vi "Demo Seq Tester.vi"() -> ()   [LabVIEW 2014]
uses:
  <vilib>/Utility/miscctls.llb/LVRowAndColumnTypeDef.ctl
  TypeDefs/STEP Display.ctl
  Mimico Display/TypeDefs/Mimic Data.ctl
  Mimico Display/TypeDefs/BG Image.ctl
  Mimico Display/TypeDefs/mObject.ctl
  02_SEQ/TypeDefs/Sequence.ctl
  02_SEQ/TypeDefs/STEP.ctl
  02_SEQ/TypeDefs/LogicParsedExpression.ctl
  02_SEQ/TypeDefs/HW InOut MAP.ctl
  02_SEQ/TypeDefs/Program.ctl
  APIs/Data Queue/Control Data Cluster.ctl
  SEQ Monitoring Global Variables.vi
  DO Monitoring Global Variables.vi
  APIs/Message Queue/Enqueue Message (Single).vi
  APIs/Message Queue/WINFAS 2 Message Queue.lvlib
  02_SEQ/SeqLoop.lvlib
  APIs/Data Queue/WINFAS 2 Data Queue.lvlib
  Mimico Display/Mimico Display.lvlib
panel:
  out "Current Prog Name":string caption="Info"
  out "Current Prog Info":string caption="Info"
  in  "MIMIC":bool
  in  "SEC":bool
  in  "HOME":bool
  in  "Tab Control":enum32{"HOME", "SEC", "MIMIC", "MESSAGE"}(tab)=enum."SEC"
  in  "New Cfg":bool
  in  "Open Cfg":bool
  in  "Save Cfg":bool
  in  "New Prog":bool
  in  "Delete Prog":bool
  in  "Config Prog":bool
  in  "I/O Config":bool
  in  "Editor de Programas":i32(listbox)=-1 caption="Secuencia"
  out "Current Sequence":string[][](table)
  in  "Angle":sgl(knob) scale=-720.0..720.0
  in  "Start Sec A-Z":bool
  in  "Start Sec Ciclo":bool
  in  "Tab Control HardW":enum32{"Hw 1", "Hw 2", "Hw 3", "Hw 4", "Hw 5"}(tab)
  in  "Conf In":T1
  in  "Conf In 2":T1
  in  "Conf In 3":T1
  in  "Conf In 4":T1
  in  "Conf In 5":T1
  in  "OutPuts":T2(tab)
  out "View Out":T3
  out "View Out 2":T3
  out "View Out 3":T3
  out "View Out 4":T3
  out "View Out 5":T3
  out "Error":bool
  out "Alarma":bool
  out "Show Main Error&Alarm":string[][](table)
  out "Acept":bool
  out "Alarms Message":string
  out "Error Message":string
  out "Operator Message":string
  out "Mimic":picture
  out "MATH":string
  out "HWAsync 10":string
  out "HWAsync 9":string
  out "HWAsync 8":string
  out "HWAsync 7":string
  out "HWAsync 6":string
  out "HWAsync 5":string
  out "HWAsync 4":string
  out "HWAsync 3":string
  out "HWAsync 2":string
  out "HWAsync 1":string
  out "HWSync 5":string
  out "DO 5":bool[](array[boolean]) caption="DO-HWSync 5 -->"
  out "HWSync 4":string
  out "DO 4":bool[](array[boolean]) caption="DO-HWSync 4 -->"
  out "HWSync 3":string
  out "DO 3":bool[](array[boolean]) caption="DO-HWSync 3 -->"
  out "HWSync 2":string
  out "DO 2":bool[](array[boolean]) caption="DO-HWSync 2 -->"
  out "HWSync 1":string
  out "DO 1":bool[](array[boolean]) caption="DO-HWSync 1 -->"
  in  "MESSAGE":bool
  in  "error in (no error)":errorcluster
  in  "Tab Control 2":enum32{"HOME", "PIC", "TAB"}(tab)=enum."PIC"
  out "Mimic Small":picture
  out "Cond. Avan.":string[][](table)
  # "DEMO - Secuencial"
  # "Lista de Programas de Medición"
  # "Editor de Programas"
  # "Instrucciones: \n1)Utilice los botones de crear o borrar programa para agregar o borrar la referencia a la \"Lista de Programas de Medición\".\n2)Utilice la opción de configuración de programas para editar o configurar el programa previamente creado o cargado.\n3)Utilice la opción de configuración de I/O para configurar todas las entradas y salidas que se deseen usar."
  # "Configuración"
  # "Secuencia de Ciclo de Medición"
  # "Estado"
  # "Encoder"
  # "Mensaje de Operador:"
  # "Alarmas:"
  # "Dispositivos SINCRONOS"
  # "Módulo MATEMATICO"
  # "Dispositivos ASINCRONOS"
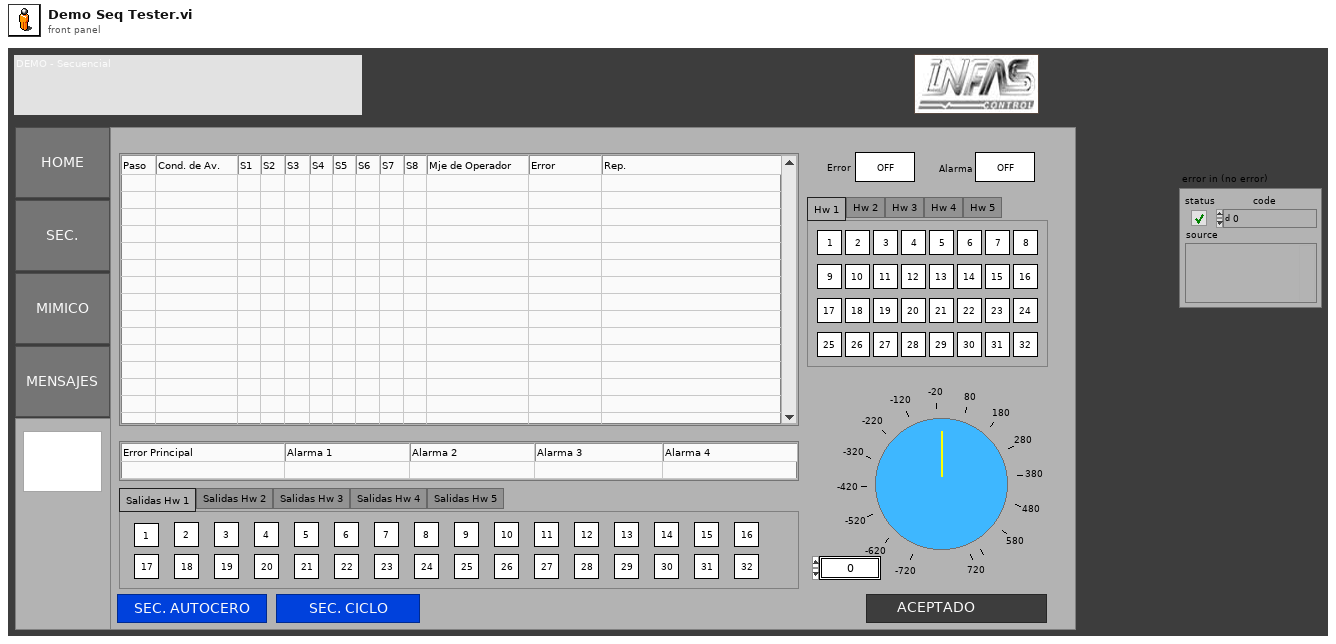
[diagram p1: front panel]
types:
  T1 = cluster{"Boolean 31":bool, "Boolean 2":bool, "Boolean 30":bool, "Boolean 29":bool, "Boolean 28":bool, "Boolean 27":bool, "Boolean 13":bool, "Boolean 14":bool, "Boolean 26":bool, "Boolean 25":bool, "Boolean 24":bool, "Boolean 23":bool, "Boolean 32":bool, "Boolean 1":bool, "Boolean 3":bool, "Boolean 4":bool, "Boolean 5":bool, "Boolean 6":bool, "Boolean 7":bool, "Boolean 8":bool, "Boolean 9":bool, "Boolean 10":bool, "Boolean 11":bool, "Boolean 12":bool, "Boolean 20":bool, "Boolean 18":bool, "Boolean 19":bool, "Boolean 17":bool, "Boolean 16":bool, "Boolean 15":bool, "Boolean 22":bool, "Boolean 21":bool}
  T2 = enum32{"Salidas Hw 1", "Salidas Hw 2", "Salidas Hw 3", "Salidas Hw 4", "Salidas Hw 5"}
  T3 = cluster{"Boolean 36":bool, "Boolean 3":bool, "Boolean 35":bool, "Boolean 34":bool, "Boolean 33":bool, "Boolean 32":bool, "Boolean 16":bool, "Boolean 17":bool, "Boolean 26":bool, "Boolean 25":bool, "Boolean 24":bool, "Boolean 23":bool, "Boolean 37":bool, "Boolean 1":bool, "Boolean 15":bool, "Boolean 4":bool, "Boolean 5":bool, "Boolean 6":bool, "Boolean 7":bool, "Boolean 8":bool, "Boolean 9":bool, "Boolean 10":bool, "Boolean 11":bool, "Boolean 12":bool, "Boolean 38":bool, "Boolean 21":bool, "Boolean 22":bool, "Boolean 20":bool, "Boolean 19":bool, "Boolean 18":bool, "Boolean 40":bool, "Boolean 39":bool}
  T4 = typedef "SeqLoop.lvlib/STEP.ctl" = cluster{"STEP N°":u32, "STEP Switch":cluster{"jump?":bool, "Initial STEP":u32, "Number of STEPs":u32, "Repetitions":u32, "Reset?":bool}, "Outputs":i32[], "STEP Check":cluster{"Advance":T5, "Error ":T5, "Alarm 1":T5, "Alarm 2":T5, "Alarm 3":T5, "Alarm 4":T5}, "Display":cluster{"Mssg Op":string, "Mimic Data":T6}}
  T5 = typedef "SeqLoop.lvlib/LogicParsedExpression.ctl" = cluster{"RPN ":string[], "Variables":string[], "Ctes":string[], "Formula":string, "Message":string}
  T6 = typedef "SeqLoop.lvlib/Mimico Display.lvlib/Mimic Data.ctl" = cluster{"BG Image":T7, "Mimic mObjects":T8[]}
  T7 = typedef "SeqLoop.lvlib/Mimico Display.lvlib/BG Image.ctl" = cluster{"Path":path, "point":cluster{"x":i16, "y":i16}}
  T8 = typedef "SeqLoop.lvlib/Mimico Display.lvlib/mObject.ctl" = cluster{"point":cluster{"x":i16, "y":i16}, "Precision (Digits)":i32, "Visible?":bool, "Ref":string, "Comment":string}
  T9 = typedef "SeqLoop.lvlib/Sequence.ctl" = cluster{"STEPs":T4[], "Main Error&Alarm":cluster{"Main Error":T5, "Main Alarm 1":T5, "Main Alarm 2":T5, "Main Alarm 3":T5, "Main Alarm 4":T5}}
  T10 = cluster{"HWS1":string, "HWS2":string, "HWS3":string, "HWS4":string, "HWS5":string, "MATH":string}
  T11 = enum8{"Enabled", "Disabled", "Disabled and Grayed Out"}
  T12 = typedef "STEP Display.ctl" = cluster{"Mimic Data":T6, "Operator Mssg":string, "Error":cluster{"true?":bool, "Message":string}, "Alarm 1":cluster{"true?":bool, "Message":string}, "Alarm 2":cluster{"true?":bool, "Message":string}, "Alarm 3":cluster{"true?":bool, "Message":string}, "Alarm 4":cluster{"true?":bool, "Message":string}}
  T13 = cluster{"File Direction":path, "Progs Data":variant}
  T14 = typedef "LVRowAndColumnTypeDef.ctl" = cluster{"Row":i32, "Column":i32}
  T15 = typedef "WINFAS 2 Data Queue.lvlib/All Data Queues Cluster.ctl" = cluster{"Queues":cluster{"ACQ HWSync1":refnum<queue>, "ACQ HWSync2":refnum<queue>, "ACQ HWSync3":refnum<queue>, "ACQ HWSync4":refnum<queue>, "ACQ HWSync5":refnum<queue>}, "Notifiers":cluster{"Control":cluster{"CTRL HWSync1":refnum<notifier>, "CTRL HWSync2":refnum<notifier>, "CTRL HWSync3":refnum<notifier>, "CTRL HWSync4":refnum<notifier>, "CTRL HWSync5":refnum<notifier>}, "Acquisition":cluster{"ACQ HWSync1":refnum<notifier>, "ACQ HWSync2":refnum<notifier>, "ACQ HWSync3":refnum<notifier>, "ACQ HWSync4":refnum<notifier>, "ACQ HWSync5":refnum<notifier>}, "Async":cluster{"ACQ HWAsync1":refnum<notifier>, "ACQ HWAsync2":refnum<notifier>, "ACQ HWAsync3":refnum<notifier>, "ACQ HWAsync4":refnum<notifier>, "ACQ HWAsync5":refnum<notifier>, "ACQ HWAsync6":refnum<notifier>, "ACQ HWAsync7":refnum<notifier>, "ACQ HWAsync8":refnum<notifier>, "ACQ HWAsync9":refnum<notifier>, "ACQ HWAsync10":refnum<notifier>}}}
  T16 = typedef "WINFAS 2 Message Queue.lvlib/All Message Queues.ctl" = cluster{"CORE":refnum<queue>, "Event UI":refnum<queue>, "Display UI":refnum<queue>, "MATH":refnum<queue>, "SEQ":refnum<queue>, "DB":refnum<queue>, "ERR":refnum<queue>, "HAL":refnum<queue>, "HWSync1":refnum<queue>, "HWSync2":refnum<queue>, "HWSync3":refnum<queue>, "HWSync4":refnum<queue>, "HWSync5":refnum<queue>, "HWAsync1":refnum<queue>, "HWAsync2":refnum<queue>, "HWAsync3":refnum<queue>, "HWAsync4":refnum<queue>, "HWAsync5":refnum<queue>, "HWAsync6":refnum<queue>, "HWAsync7":refnum<queue>, "HWAsync8":refnum<queue>, "HWAsync9":refnum<queue>, "HWAsync10":refnum<queue>}
  T17 = cluster{"CTRL HWSync1":refnum<notifier>, "CTRL HWSync2":refnum<notifier>, "CTRL HWSync3":refnum<notifier>, "CTRL HWSync4":refnum<notifier>, "CTRL HWSync5":refnum<notifier>}
  T18 = cluster{"File Direction":path, "Progs Data":variant}[]
  T19 = cluster{"Main Error":T5, "Main Alarm 1":T5, "Main Alarm 2":T5, "Main Alarm 3":T5, "Main Alarm 4":T5}
  T20 = enum16{"open", "replace", "create", "open or create", "replace or create", "replace or create with confirmation"}
  T21 = typedef "SeqLoop.lvlib/HW InOut MAP.ctl" = cluster{"Inputs":cluster{"Entrada":i32, "Descripción":string, "Habilitada?":bool}[][], "Outputs":cluster{"Salida":i32, "Descripción":string, "Habilitada?":bool, "Formula":string, "Tipo de Salida":string}[][]}
  T22 = typedef "SeqLoop.lvlib/Program.ctl" = cluster{"Prog. Data":cluster{"Operación":i32, "Pieza":i32, "Descripción":string, "Nombre Programa":string, "Autor":string, "Diseño":string, "Total Meds.:":i32, "Total Meds. Aux.:":i32}, "All Sequences":cluster{"Measurement":T9, "AutoZero":T9}}
  T23 = cluster{cluster{"File Direction":path, "Progs Data":variant}[]}
  T24 = typedef "WINFAS 2 Data Queue.lvlib/Control Data Cluster.ctl" = cluster{"Encoder":sgl, "DI":bool[], "DO":bool[]}
  T25 = cluster{"format string":string, "Measurement Index":i32[]}
  T26 = cluster{"MAX(T) or MIN (F)?":bool, "Mastering TDX Index":i32[]}
  T27 = enum32{"invalid app kind", "Development System", "Run Time System", "Student Edition", "Embedded LabVIEW", "Evaluation", "Custom"}
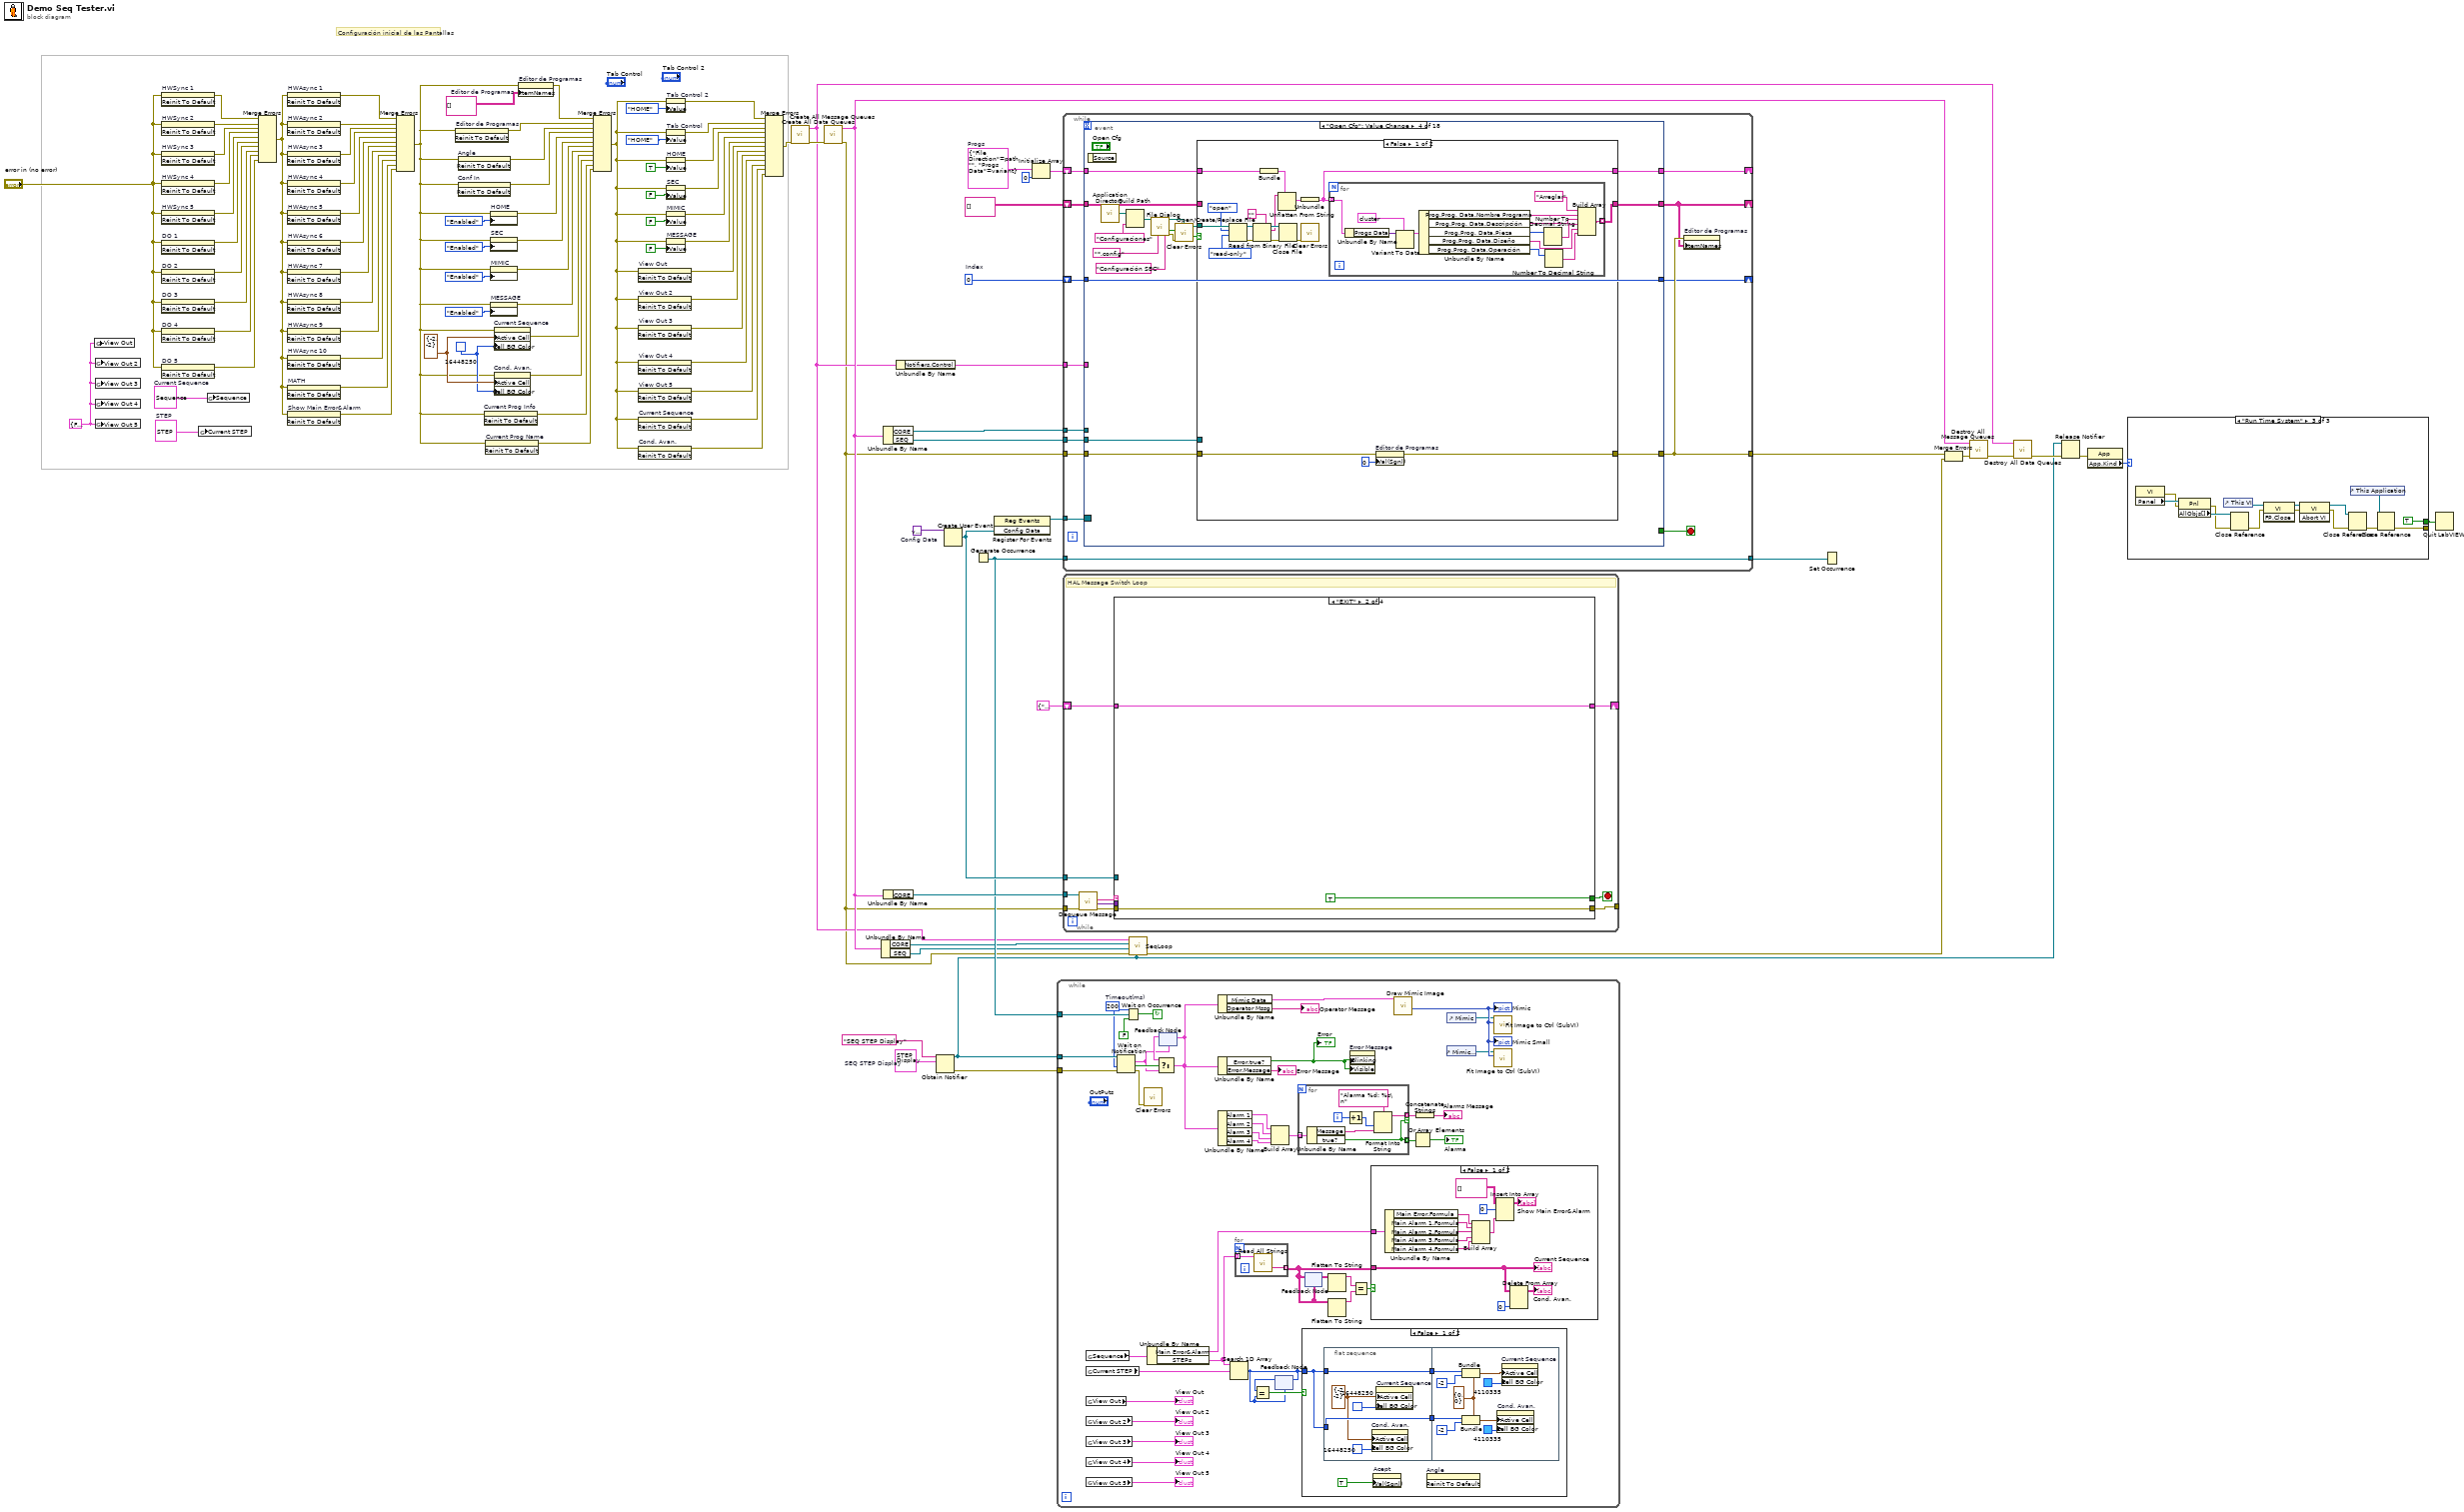
[diagram p0: block diagram]
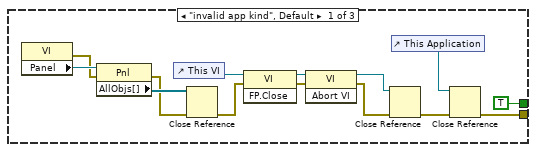
[diagram p4: hidden frame]
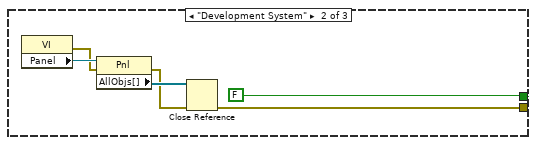
[diagram p5: hidden frame]
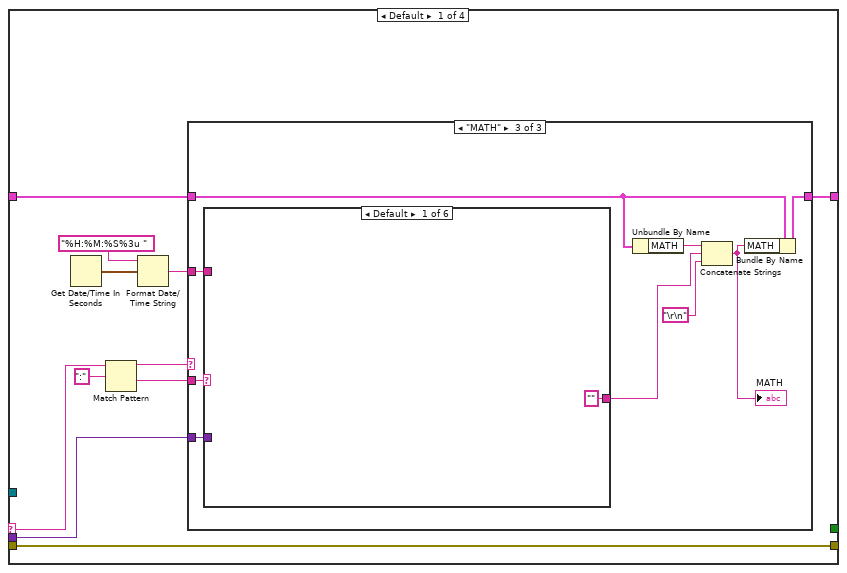
[diagram p6: hidden frame]
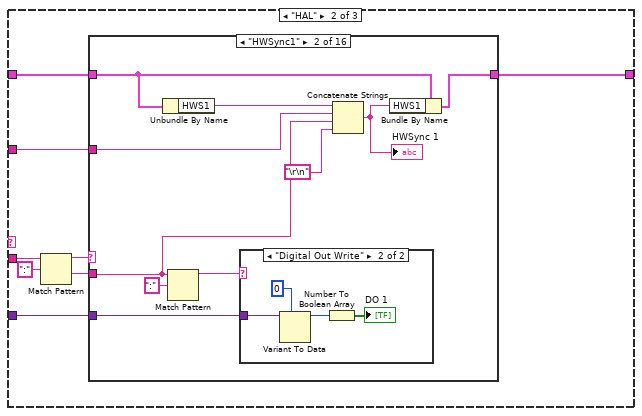
[diagram p8: hidden frame]
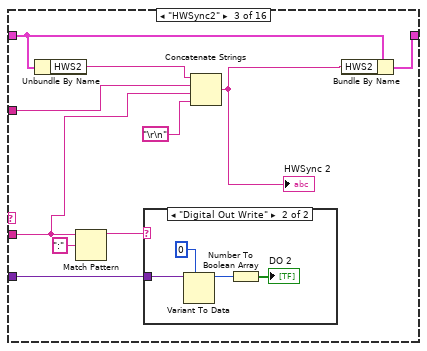
[diagram p11: hidden frame]
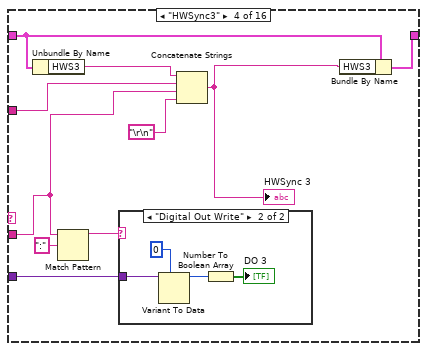
[diagram p13: hidden frame]
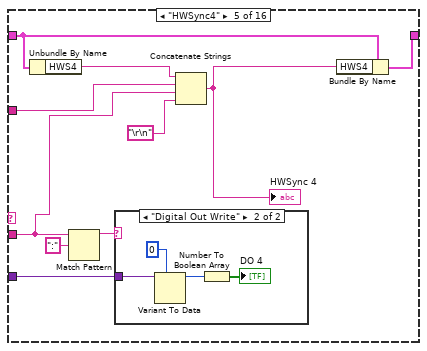
[diagram p15: hidden frame]
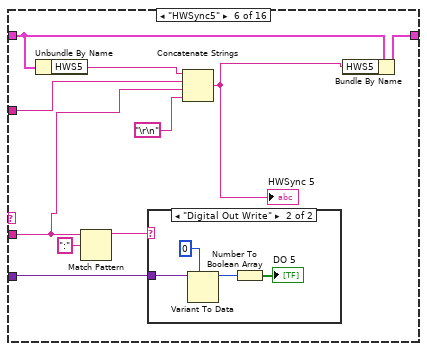
[diagram p17: hidden frame]
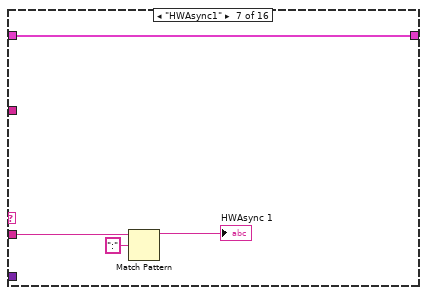
[diagram p19: hidden frame]
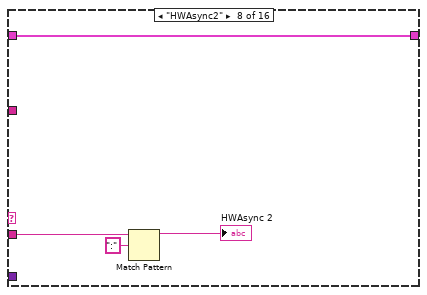
[diagram p20: hidden frame]
diagram:
  w1 = T4 {"STEP N°"=0, "STEP Switch"={"jump?"=FALSE, "Initial STEP"=0, "Number of STEPs"=0, "Repetitions"=0, "Reset?"=FALSE}, "Outputs"=[], "STEP Check"={"Advance"={"RPN "=[], "Variables"=[], "Ctes"=[], "Formula"="", "Message"=""}, "Error "={"RPN "=[], "Variables"=[], "Ctes"=[], "Formula"="", "Message"=""}, "Alarm 1"={"RPN "=[], "Variables"=[], "Ctes"=[], "Formula"="", "Message"=""}, "Alarm 2"={"RPN "=[], "Variables"=[], "Ctes"=[], "Formula"="", "Message"=""}, "Alarm 3"={"RPN "=[], "Variables"=[], "Ctes"=[], "Formula"="", "Message"=""}, "Alarm 4"={"RPN "=[], "Variables"=[], "Ctes"=[], "Formula"="", "Message"=""}}, "Display"={"Mssg Op"="", "Mimic Data"={"BG Image"={"Path"=path "", "point"={"x"=0, "y"=0}}, "Mimic mObjects"=[]}}}  # STEP
  w2 = T3 {"Boolean 36"=FALSE, "Boolean 3"=FALSE, "Boolean 35"=FALSE, "Boolean 34"=FALSE, "Boolean 33"=FALSE, "Boolean 32"=FALSE, "Boolean 16"=FALSE, "Boolean 17"=FALSE, "Boolean 26"=FALSE, "Boolean 25"=FALSE, "Boolean 24"=FALSE, "Boolean 23"=FALSE, "Boolean 37"=FALSE, "Boolean 1"=FALSE, "Boolean 15"=FALSE, "Boolean 4"=FALSE, "Boolean 5"=FALSE, "Boolean 6"=FALSE, "Boolean 7"=FALSE, "Boolean 8"=FALSE, "Boolean 9"=FALSE, "Boolean 10"=FALSE, "Boolean 11"=FALSE, "Boolean 12"=FALSE, "Boolean 38"=FALSE, "Boolean 21"=FALSE, "Boolean 22"=FALSE, "Boolean 20"=FALSE, "Boolean 19"=FALSE, "Boolean 18"=FALSE, "Boolean 40"=FALSE, "Boolean 39"=FALSE} ("View Out")
  w6 = T9 {"STEPs"=[], "Main Error&Alarm"={"Main Error"={"RPN "=[], "Variables"=[], "Ctes"=[], "Formula"="", "Message"=""}, "Main Alarm 1"={"RPN "=[], "Variables"=[], "Ctes"=[], "Formula"="", "Message"=""}, "Main Alarm 2"={"RPN "=[], "Variables"=[], "Ctes"=[], "Formula"="", "Message"=""}, "Main Alarm 3"={"RPN "=[], "Variables"=[], "Ctes"=[], "Formula"="", "Message"=""}, "Main Alarm 4"={"RPN "=[], "Variables"=[], "Ctes"=[], "Formula"="", "Message"=""}}}  # Current Sequence
  w52 = T12 {"Mimic Data"={"BG Image"={"Path"=path "", "point"={"x"=0, "y"=0}}, "Mimic mObjects"=[]}, "Operator Mssg"="", "Error"={"true?"=FALSE, "Message"=""}, "Alarm 1"={"true?"=FALSE, "Message"=""}, "Alarm 2"={"true?"=FALSE, "Message"=""}, "Alarm 3"={"true?"=FALSE, "Message"=""}, "Alarm 4"={"true?"=FALSE, "Message"=""}}  # SEQ STEP Display
  w70 = T13 {"File Direction"=path "", "Progs Data"=variant}  # Progs
  w44 = T14 {"Row"=-2, "Column"=-2} ("Active Cell:Active Cell")
  w43 = u32 16448250
  w73 = string[][] []  # Editor de Programas
  w87 = 0  # Index
  w96 = variant  # Config Data
  # "Configuración inicial de las Pantallas"
  n1 = global write "DO Monitoring Global Variables.vi" "View Out"(w2) -> ()
  n2 = global write "DO Monitoring Global Variables.vi" "View Out 2"(w2) -> ()
  n3 = global write "DO Monitoring Global Variables.vi" "View Out 3"(w2) -> ()
  n4 = global write "DO Monitoring Global Variables.vi" "View Out 4"(w2) -> ()
  n5 = global write "DO Monitoring Global Variables.vi" "View Out 5"(w2) -> ()
  n6 = invoke on="HWSync 1" class="Str" method="Reinit To Default"(error in="error in (no error)") -> (error out=w22:errorcluster)  [unwired: 2 in, 2 out]
  n7 = invoke on="HWSync 2" class="Str" method="Reinit To Default"(error in="error in (no error)") -> (error out=w21:errorcluster)  [unwired: 2 in, 2 out]
  n8 = invoke on="HWSync 3" class="Str" method="Reinit To Default"(error in="error in (no error)") -> (error out=w20:errorcluster)  [unwired: 2 in, 2 out]
  n9 = invoke on="HWSync 4" class="Str" method="Reinit To Default"(error in="error in (no error)") -> (error out=w19:errorcluster)  [unwired: 2 in, 2 out]
  n10 = invoke on="HWSync 5" class="Str" method="Reinit To Default"(error in="error in (no error)") -> (error out=w18:errorcluster)  [unwired: 2 in, 2 out]
  n11 = invoke on="DO 1" class="Arr (strict)" method="Reinit To Default"(error in="error in (no error)") -> (error out=w17:errorcluster)  [unwired: 2 in, 2 out]
  n12 = invoke on="DO 2" class="Arr (strict)" method="Reinit To Default"(error in="error in (no error)") -> (error out=w16:errorcluster)  [unwired: 2 in, 2 out]
  n13 = invoke on="DO 3" class="Arr (strict)" method="Reinit To Default"(error in="error in (no error)") -> (error out=w15:errorcluster)  [unwired: 2 in, 2 out]
  n14 = invoke on="DO 4" class="Arr (strict)" method="Reinit To Default"(error in="error in (no error)") -> (error out=w14:errorcluster)  [unwired: 2 in, 2 out]
  n15 = invoke on="DO 5" class="Arr (strict)" method="Reinit To Default"(error in="error in (no error)") -> (error out=w13:errorcluster)  [unwired: 2 in, 2 out]
  n16 = global write "SEQ Monitoring Global Variables.vi" "Current STEP"(w1) -> ()
  n17 = global write "SEQ Monitoring Global Variables.vi" "Sequence"(w6) -> ()
  n18 = Merge Errors(w22, w21, w20, w19, w18, w17, w16, w15, w14, w13) -> (w4:errorcluster)
  n19 = invoke on="HWAsync 1" class="Str" method="Reinit To Default"(error in=w4) -> (error out=w33:errorcluster)  [unwired: 2 in, 2 out]
  n20 = invoke on="HWAsync 2" class="Str" method="Reinit To Default"(error in=w4) -> (error out=w32:errorcluster)  [unwired: 2 in, 2 out]
  n21 = invoke on="HWAsync 3" class="Str" method="Reinit To Default"(error in=w4) -> (error out=w31:errorcluster)  [unwired: 2 in, 2 out]
  n22 = invoke on="HWAsync 4" class="Str" method="Reinit To Default"(error in=w4) -> (error out=w30:errorcluster)  [unwired: 2 in, 2 out]
  n23 = invoke on="HWAsync 5" class="Str" method="Reinit To Default"(error in=w4) -> (error out=w29:errorcluster)  [unwired: 2 in, 2 out]
  n24 = invoke on="HWAsync 6" class="Str" method="Reinit To Default"(error in=w4) -> (error out=w28:errorcluster)  [unwired: 2 in, 2 out]
  n25 = invoke on="HWAsync 7" class="Str" method="Reinit To Default"(error in=w4) -> (error out=w27:errorcluster)  [unwired: 2 in, 2 out]
  n26 = invoke on="HWAsync 8" class="Str" method="Reinit To Default"(error in=w4) -> (error out=w26:errorcluster)  [unwired: 2 in, 2 out]
  n27 = invoke on="HWAsync 9" class="Str" method="Reinit To Default"(error in=w4) -> (error out=w25:errorcluster)  [unwired: 2 in, 2 out]
  n28 = invoke on="HWAsync 10" class="Str" method="Reinit To Default"(error in=w4) -> (error out=w24:errorcluster)  [unwired: 2 in, 2 out]
  n29 = invoke on="MATH" class="Str" method="Reinit To Default"(error in=w4) -> (error out=w23:errorcluster)  [unwired: 2 in, 2 out]
  n30 = invoke on="Show Main Error&Alarm" class="Tbl (strict)" method="Reinit To Default"(error in=w4) -> (error out=w5:errorcluster)  [unwired: 2 in, 2 out]
  n31 = Merge Errors(w33, w32, w31, w30, w29, w28, w27, w26, w25, w24, w23, w5) -> (w11:errorcluster)
  n32 = invoke on="Editor de Programas" class="MCListbox (strict)" method="Reinit To Default"(error in=w11) -> (error out=w54:errorcluster)  [unwired: 2 in, 2 out]
  n33 = invoke on="Angle" class="Knob (strict)" method="Reinit To Default"(error in=w11) -> (error out=w99:errorcluster)  [unwired: 2 in, 2 out]
  n34 = invoke on="Conf In" class="Clust (strict)" method="Reinit To Default"(error in=w11) -> (error out=w100:errorcluster)  [unwired: 2 in, 2 out]
  n35 = invoke on="Current Prog Info" class="Str" method="Reinit To Default"(error in=w11) -> (error out=w39:errorcluster)  [unwired: 2 in, 2 out]
  n36 = invoke on="Current Prog Name" class="Str" method="Reinit To Default"(error in=w11) -> (error out=w10:errorcluster)  [unwired: 2 in, 2 out]
  n37 = property on="HOME" class="Bool (strict)"(error in=w11, "DisabledEnum"=T11."Enabled" ("Disabled")) -> (error out=w77:errorcluster)  [unwired: 1 in, 1 out]
  n38 = property on="SEC" class="Bool (strict)"(error in=w11, "DisabledEnum"=T11."Enabled" ("Disabled")) -> (error out=w68:errorcluster)  [unwired: 1 in, 1 out]
  n39 = property on="MIMIC" class="Bool (strict)"(error in=w11, "DisabledEnum"=T11."Enabled" ("Disabled")) -> (error out=w67:errorcluster)  [unwired: 1 in, 1 out]
  n40 = property on="MESSAGE" class="Bool (strict)"(error in=w11, "DisabledEnum"=T11."Enabled" ("Disabled")) -> (error out=w45:errorcluster)  [unwired: 1 in, 1 out]
  n41 = property on="Current Sequence" class="Tbl (strict)"(error in=w11, "Active Cell"=w44, "Cell BG Color"=w43) -> (error out=w46:errorcluster)  [unwired: 1 in, 1 out]
  n42 = property on="Cond. Avan." class="Tbl (strict)"(error in=w11, "Active Cell"=w44, "Cell BG Color"=w43) -> (error out=w42:errorcluster)  [unwired: 1 in, 1 out]
  n43 = property on="Editor de Programas" class="MCListbox (strict)"(error in=w11, "ItemNames"=w73) -> (error out=w53:errorcluster)  [unwired: 1 in, 1 out]
  n44 = Merge Errors(w53, w54, w99, w100, w77, w68, w67, w45, w46, w42, w39, w10) -> (w9:errorcluster)
  n45 = invoke on="View Out" class="Clust (strict)" method="Reinit To Default"(error in=w9) -> (error out=w38:errorcluster)  [unwired: 2 in, 2 out]
  n46 = invoke on="View Out 2" class="Clust (strict)" method="Reinit To Default"(error in=w9) -> (error out=w37:errorcluster)  [unwired: 2 in, 2 out]
  n47 = invoke on="View Out 3" class="Clust (strict)" method="Reinit To Default"(error in=w9) -> (error out=w36:errorcluster)  [unwired: 2 in, 2 out]
  n48 = invoke on="View Out 4" class="Clust (strict)" method="Reinit To Default"(error in=w9) -> (error out=w35:errorcluster)  [unwired: 2 in, 2 out]
  n49 = invoke on="View Out 5" class="Clust (strict)" method="Reinit To Default"(error in=w9) -> (error out=w34:errorcluster)  [unwired: 2 in, 2 out]
  n50 = invoke on="Current Sequence" class="Tbl (strict)" method="Reinit To Default"(error in=w9) -> (error out=w8:errorcluster)  [unwired: 2 in, 2 out]
  n51 = invoke on="Cond. Avan." class="Tbl (strict)" method="Reinit To Default"(error in=w9) -> (error out=w7:errorcluster)  [unwired: 2 in, 2 out]
  n52 = property on="Tab Control 2" class="TabCtl (strict)"(error in=w9, "Value"=enum32{"HOME", "PIC", "TAB"}."HOME" ("Tab Control 2")) -> (error out=w41:errorcluster)  [unwired: 1 in, 1 out]
  n53 = property on="Tab Control" class="TabCtl (strict)"(error in=w9, "Value"=enum32{"HOME", "SEC", "MIMIC", "MESSAGE"}."HOME" ("Tab Control")) -> (error out=w76:errorcluster)  [unwired: 1 in, 1 out]
  n54 = property on="HOME" class="Bool (strict)"(error in=w9, "Value"=TRUE ("HOME")) -> (error out=w75:errorcluster)  [unwired: 1 in, 1 out]
  n55 = property on="SEC" class="Bool (strict)"(error in=w9, "Value"=FALSE ("CICLO")) -> (error out=w74:errorcluster)  [unwired: 1 in, 1 out]
  n56 = property on="MIMIC" class="Bool (strict)"(error in=w9, "Value"=FALSE ("CONFIG.")) -> (error out=w66:errorcluster)  [unwired: 1 in, 1 out]
  n57 = property on="MESSAGE" class="Bool (strict)"(error in=w9, "Value"=FALSE ("CONFIG.")) -> (error out=w49:errorcluster)  [unwired: 1 in, 1 out]
  n58 = Merge Errors(w41, w76, w75, w74, w66, w49, w38, w37, w36, w35, w34, w8, w7) -> (w65:errorcluster)
  n59 = call "Create All Data Queues.vi"("Error In"=w65) -> ("Error Out"=w64:errorcluster, "WINFAS 2 Data Queue.lvlib:All Data Queues Cluster"=w57:T15)  [unwired: 9 in]
  n60 = call "Create All Message Queues.vi"("error in (no error)"=w64) -> ("error out"=w56:errorcluster, "Message Queues Out"=w61:T16)  [unwired: 9 in]
  n61 = Unbundle By Name(w61) -> ("CORE"=w59:refnum<queue>, "SEQ"=w58:refnum<queue>)
  n62 = Unbundle By Name(w61) -> ("CORE"=w92:refnum<queue>, "SEQ"=w93:refnum<queue>)
  n63 = Unbundle By Name(w61) -> ("CORE"=w97:refnum<queue>)
  n64 = Unbundle By Name(w57) -> ("Notifiers.Control"=w60:T17)
  n65 = Obtain Notifier(name (unnamed)="SEQ STEP Display", notification data type=w52) -> (notifier out=w51:refnum<notifier>, error out=w83:errorcluster)  [unwired: 2 in, 1 out]
  n66 = Create User Event(user event datatype=w96) -> (user event=w94:refnum<user-event>)  [unwired: 1 in, 1 out]
  n67 = Generate Occurrence() -> (w81:refnum<k4>)
  n68 = register-events(w94) -> (reference out=w95:refnum<event-registration>)  [unwired: 2 in, 1 out]
  n69 = Initialize Array(w70, 0 ("dimension size")) -> (w71:T18)
  n70 = while {
    tunnel: w51 -> [w145]
    tunnel: w83 -> [w140]
    tunnel: w81 -> [w138]
    stop <- w139 continue-if-true
    w136 = 200  # Timeout(ms)
    n71 = global read "SEQ Monitoring Global Variables.vi" "Sequence"() -> (w109:T9)
    n72 = global read "SEQ Monitoring Global Variables.vi" "Current STEP"() -> (w119:T4)
    n73 = global read "DO Monitoring Global Variables.vi" "View Out"() -> (→"View Out":T3)
    n74 = global read "DO Monitoring Global Variables.vi" "View Out 2"() -> (→"View Out 2":T3)
    n75 = global read "DO Monitoring Global Variables.vi" "View Out 3"() -> (→"View Out 3":T3)
    n76 = global read "DO Monitoring Global Variables.vi" "View Out 4"() -> (→"View Out 4":T3)
    n77 = global read "DO Monitoring Global Variables.vi" "View Out 5"() -> (→"View Out 5":T3)
    n78 = Wait on Notification(notifier=w145, timeout in ms (-1)=w136, error in (no error)=w140) -> (notification=w137:T12, timed out?=w144:bool, error out=w142:errorcluster)  [unwired: 1 in, 1 out]
    n79 = Wait on Occurrence(1:FALSE ("ignore previous (T)"), 2:w138, 3:w136) -> (0:w139:bool)
    n80 = call <vilib>:"Clear Errors.vi"("error in (no error)"=w142) -> ()  [unwired: 5 in, 2 out]
    n81 = Unbundle By Name(w109) -> ("Main Error&Alarm"=w102:T19, "STEPs"=w108:T4[])
    n82 = feedback #1(w137) -> (w143:T12)
    n83 = Select(t=w143, s=w144, f=w137) -> (s? t:f=w129:T12)
    n84 = feedback-in #1(w129) -> ()
    n85 = Unbundle By Name(w129) -> ("Mimic Data"=w132:T6, "Operator Mssg"=→"Operator Message":string)
    n86 = Unbundle By Name(w129) -> ("Error.true?"=w110:bool, "Error.Message"=→"Error Message":string)
    "Error" <- w110
    n87 = Unbundle By Name(w129) -> ("Alarm 1"=w128:cluster{"true?":bool, "Message":string}, "Alarm 2"=w127:cluster{"true?":bool, "Message":string}, "Alarm 3"=w126:cluster{"true?":bool, "Message":string}, "Alarm 4"=w125:cluster{"true?":bool, "Message":string})
    n88 = Search 1D Array(1D array=w108, element=w119) -> (index of element=w118:i32)  [unwired: 1 in]
    n89 = for {
      tunnel: w108 -> [w178] mode=indexing
      tunnel: [w177] -> w103 mode=indexing
      n90 = call "Read All Strings.vi"("STEP in"=w178) -> ("All Strings"=w177:string[])  [unwired: 8 in, 2 out]
    }
    n91 = Build Array(w128, w127, w126, w125) -> (w124:cluster{"true?":bool, "Message":string}[])
    n92 = feedback #2(w118) -> (w121:i32)
    n93 = Equal?(x=w121, y=w118) -> (x = y?=w120:bool)
    n94 = feedback-in #2(w118) -> ()
    n95 = for {
      tunnel: w124 -> [w185] mode=indexing
      tunnel: [w180] -> w123 mode=indexing if=w179
      tunnel: [w179] -> w112 mode=indexing
      i -> [w183]
      n96 = Unbundle By Name(w185) -> ("Message"=w181:string, "true?"=w179:bool)
      n97 = Increment(x=w183) -> (x+1=w182:i32)
      n98 = Format Into String(format string="Alarma %d: %s\n", w182, w181) -> (resulting string=w180:string)  [unwired: 2 in, 1 out]
    }
    n99 = case shown="False" w120 {
      tunnel: w118 -> [w160 _]
      frame False {
        n100 = flat-sequence {
          tunnel: w160 -> [w167]
          tunnel: [w167] -> w162
          tunnel: [w164] -> w161
          tunnel: w160 -> [w164]
          tunnel: w162 -> [w173]
          tunnel: w161 -> [w172]
          frame #0 {
            w163 = T14 {"Row"=-2, "Column"=-2} ("Active Cell:Active Cell")
            n101 = property on="Cond. Avan." class="Tbl (strict)"("Active Cell"=w163, "Cell BG Color"=u32 16448250) -> ()  [unwired: 2 in, 2 out]
            n102 = property on="Current Sequence" class="Tbl (strict)"("Active Cell"=w163, "Cell BG Color"=u32 16448250) -> ()  [unwired: 2 in, 2 out]
          }
          frame #1 {
            w168 = cluster{i32, "Row":i32} {0, "Row"=0} ("output cluster")
            n103 = Bundle(cluster=w168, w173, "Row"=-2) -> (w175:cluster{i32, "Row":i32})
            n104 = Bundle(cluster=w168, w172, "Row"=-2) -> (w170:cluster{i32, "Row":i32})
            n105 = property on="Cond. Avan." class="Tbl (strict)"("Active Cell"=w170, "Cell BG Color"=u32 4110335) -> ()  [unwired: 2 in, 2 out]
            n106 = property on="Current Sequence" class="Tbl (strict)"("Active Cell"=w175, "Cell BG Color"=u32 4110335) -> ()  [unwired: 2 in, 2 out]
          }
        }
        n107 = property on="Acept" class="Bool"("Val(Sgnl)"=TRUE) -> ()  [unwired: 2 in, 2 out]
        n108 = invoke on="Angle" class="Knob (strict)" method="Reinit To Default"() -> ()  [unwired: 3 in, 3 out]
      }
      frame True {
      }
    }
    n109 = feedback #3(w103) -> (w107:string[][])
    n110 = feedback-in #3(w103) -> ()
    n111 = Flatten To String(anything=w107) -> (data string=w106:string)  [unwired: 3 in, 2 out]
    n112 = Flatten To String(anything=w103) -> (data string=w105:string)  [unwired: 3 in, 2 out]
    n113 = property on="Error Message" class="Str"("Blinking"=w110, "Visible"=w110) -> ()  [unwired: 2 in, 2 out]
    n114 = Equal?(x=w106, y=w105) -> (x = y?=w104:bool)
    n115 = case shown="False" w104 {
      tunnel: w103 -> [w156 _]
      tunnel: w102 -> [w152 _]
      frame False {
        n116 = Unbundle By Name(w152) -> ("Main Error.Formula"=w150:string, "Main Alarm 1.Formula"=w149:string, "Main Alarm 2.Formula"=w151:string, "Main Alarm 3.Formula"=w148:string, "Main Alarm 4.Formula"=w147:string)
        n117 = Build Array(w150, w149, w151, w148, w147) -> (w146:string[])
        n118 = Insert Into Array(array=string[][] [] ("Show Main Error&Alarm 2"), index (row)=0, new element=w146) -> (→"Show Main Error&Alarm":string[][])  [unwired: 1 in]
        n119 = Delete From Array(array=w156, index (col)=0 ("disabled index (col)")) -> (array with subset deleted=→"Cond. Avan.":string[][])  [unwired: 2 in, 1 out]
        "Current Sequence" <- w156
      }
      frame True {
      }
    }
    n120 = call "Draw Mimic Image.vi"("Mimic Data in"=w132) -> ("Mimic Picture"=w135:picture)  [unwired: 10 in]
    "Mimic" <- w135
    "Mimic Small" <- w135
    n121 = Or Array Elements(Boolean array=w112) -> (logical OR=→"Alarma":bool)
    n122 = Concatenate Strings(w123) -> (→"Alarms Message":string)
    n123 = control-ref of="Mimic"() -> (w134:refnum<vi>)
    n124 = control-ref of="Mimic Small"() -> (w133:refnum<vi>)
    n125 = call "Fit Image to Ctrl (SubVI).vi"("picture in"=w135, "Picture ref in"=w134) -> ()  [unwired: 10 in]
    n126 = call "Fit Image to Ctrl (SubVI).vi"("picture in"=w135, "Picture ref in"=w133) -> ()  [unwired: 10 in]
  }
  n127 = while {
    tunnel: w56 -> [w199]
    tunnel: [w193] -> w101
    tunnel: w95 -> [w197]
    tunnel: w93 -> [w196]
    tunnel: w92 -> [w195]
    shift-right: [w192] -> _
    shift-left: w87 -> [w194]
    tunnel: w81 -> [w191]
    tunnel: [w191] -> w82
    shift-right: [w189] -> _
    shift-left: w71 -> [w190]
    shift-right: [w187] -> _
    shift-left: string[][] [] -> [w188]
    tunnel: w60 -> [w186]
    stop <- w198 stop-if-true
    n128 = event shown="[3] \"Open Cfg\": Value Change" {
      selector: w197 -> [_ _ _ _ _ _ _ _ _ _ _ _ _ _ _ _ _ _]
      dyn-events: _ -> [_ _ _ _ _ _ _ _ _ _ _ _ _ _ _ _ _ _]
      timeout: _ -> [_ _ _ _ _ _ _ _ _ _ _ _ _ _ _ _ _ _]
      tunnel: w199 -> [w216 w230 w252 w291 w338 w360 w390 w412 w435 w460 w482 w497 w504 w527 w548 w569 w610 w638]
      tunnel: [w221 w226 w268 w289 w337 w385 w406 w434 w454 w467 w480 w498 w518 w525 w546 w567 w604 w636] -> w193
      tunnel: [_ _ _ _ _ _ _ _ _ _ _ _ _ _ _ _ _ TRUE ("Discard?")] -> w198
      tunnel: w196 -> [w223 _ w253 w292 _ w362 _ _ _ _ w483 w496 _ w544 w564 _ _ w634]
      tunnel: w195 -> [_ _ _ _ _ _ _ _ _ _ _ _ _ w526 w547 _ _ w635]
      tunnel: ["Editor de Programas" w233 w256 w302 _ w369 w402 w413 w452 _ w485 w493 w513 w542 w563 w566 w628 w633] -> w192
      tunnel: w194 -> [_ w235 w259 w302 _ w363 w402 w413 w452 _ w485 w493 w513 w542 w563 w566 w628 w633]
      tunnel: w190 -> [w225 w229 w261 w293 w340 w364 w401 w427 w448 w479 w484 w495 w520 w541 w562 w572 w630 w632]
      tunnel: [w225 w228 w260 w290 w340 w370 w401 w427 w448 w479 w484 w495 w519 w541 w562 w572 w630 w632] -> w189
      tunnel: w188 -> [w200 w232 w258 w287 w339 w386 w400 w414 w444 w478 w489 w494 w516 w540 w561 w571 w629 w631]
      tunnel: [w200 w231 w257 w288 w339 w387 w400 w414 w444 w478 w489 w494 w515 w540 w561 w571 w629 w631] -> w187
      tunnel: w186 -> [_ _ _ _ _ _ _ _ _ _ _ _ _ _ _ _ w603 _]
      event "Editor de Programas": Value Change {
        w215 = T14 {"Row"=-2, "Column"=-2} ("Active Cell:Active Cell")
        w214 = u32 16448250
        n129 = event-data() -> ()  [unwired: 1 in, 1 out]
        n130 = property on="Current Sequence" class="Tbl (strict)"(error in=w216, "Active Cell"=w215, "Cell BG Color"=w214) -> (error out=w212:errorcluster)  [unwired: 1 in, 1 out]
        n131 = property on="Cond. Avan." class="Tbl (strict)"(error in=w216, "Active Cell"=w215, "Cell BG Color"=w214) -> (error out=w213:errorcluster)  [unwired: 1 in, 1 out]
        n132 = Index Array(array=w200, index (row) #1="Editor de Programas", index (col) #1=1 ("disabled index (col)"), index (row) #2="Editor de Programas", index (col) #2=0 ("disabled index (col)"), index (row) #3="Editor de Programas", index (col) #3=2 ("index (row)"), index (row) #4="Editor de Programas", index (col) #4=6 ("index (col)")) -> (element #1=w203:string, element #2=w210:string, element #3=w209:string, element #4=w208:string)
        n133 = Merge Errors(w212, w213) -> (w211:errorcluster)
        n134 = Index Array(array=w225, index="Editor de Programas") -> (element=w222:T13)
        n135 = Unbundle By Name(w222) -> ("Progs Data"=w217:variant)
        n136 = Concatenate Strings("Nombre Programa: ", w203) -> (→"Current Prog Name":string)
        n137 = call-poly "Enqueue Message.vi"("error in (no error)"=w211, "Message Data"=w217, "Message"="Config:Set" ("Cmd String"), "Message Queue"=w223) -> ("error out"=w221:errorcluster)  [unwired: 6 in, 1 out]
        n138 = Format Into String(format string="COD. Prog. : %s - Descripción: %s - Tipo de Prog.: %s", w210, w209, w208) -> (resulting string=→"Current Prog Info":string)  [unwired: 2 in, 1 out]
      }
      event "Delete Prog": Value Change {
        n139 = event-data() -> ()  [unwired: 1 in, 1 out]
        n140 = Increment(x=w235) -> (x+1=w236:i32)
        n141 = Number To Decimal String(number=w236) -> (decimal integer string=w238:string)  [unwired: 1 in]
        n142 = Concatenate Strings("Desea Borrar el elemento: " ("message"), w238) -> (w237:string)
        n143 = Two Button Dialog(message=w237) -> (T button?=w234:bool)  [unwired: 2 in]
        n144 = case shown="False" w234 {
          tunnel: [w243 w249] -> w231
          tunnel: w232 -> [w243 w248]
          tunnel: w235 -> [w242 w244]
          tunnel: w230 -> [w241 w247]
          tunnel: [w241 w247] -> w227
          tunnel: [w242 w244] -> w233
          tunnel: w229 -> [w240 w246]
          tunnel: [w240 w245] -> w228
          frame False {
          }
          frame True {
            n145 = Delete From Array(array=w246, index=w244) -> (array with subset deleted=w245:T18)  [unwired: 1 in, 1 out]
            n146 = Delete From Array(array=w248, index (row)=w244) -> (array with subset deleted=w249:string[][])  [unwired: 2 in, 1 out]
          }
        }
        n147 = invoke on="Current Prog Info" class="Str" method="Reinit To Default"(error in=w227) -> (error out=w226:errorcluster)  [unwired: 2 in, 2 out]
      }
      event "New Cfg": Value Change {
        w255 = T13 {"File Direction"=path "", "Progs Data"=variant}  # Progs
        n148 = event-data() -> ()  [unwired: 1 in, 1 out]
        n149 = Initialize Array(w255, 15 ("dimension size")) -> (w264:T18)
        n150 = Flatten To String(anything=w264) -> (data string=w266:string)  [unwired: 3 in, 2 out]
        n151 = Flatten To String(anything=w261) -> (data string=w265:string)  [unwired: 3 in, 2 out]
        n152 = Not Equal?(x=w265, y=w266) -> (x != y?=w267:bool)
        n153 = case "Algún Prog cargado?" shown="True" w267 {
          tunnel: [TRUE ("T button?") w273] -> w262
          frame False {
          }
          frame True {
            n154 = Two Button Dialog(message="Desea crear una nueva lista de Programas?\n(Se descargarán todos los Programas cargados)") -> (T button?=w273:bool)  [unwired: 2 in]
          }
        }
        n155 = case shown="False" w262 {
          tunnel: [w277 w285] -> w260
          tunnel: w261 -> [w277 _]
          tunnel: w259 -> [w275 _]
          tunnel: w258 -> [w276 _]
          tunnel: [w276 string[][] []] -> w257
          tunnel: [w275 0 ("Index")] -> w256
          tunnel: w253 -> [_ w280]
          tunnel: w252 -> [w274 w279]
          tunnel: [w274 w278] -> w250
          frame False {
          }
          frame True {
            w282 = T13 {"File Direction"=path "", "Progs Data"=variant}  # Progs
            n156 = call-poly "Enqueue Message.vi"("error in (no error)"=w279, "Message"="INIT" ("Cmd String"), "Message Queue"=w280) -> ("error out"=w278:errorcluster)  [unwired: 7 in, 1 out]
            n157 = Initialize Array(w282, 0 ("dimension size")) -> (w285:T18)
          }
        }
        n158 = invoke on="Angle" class="Knob (strict)" method="Reinit To Default"(error in=w250) -> (error out=w269:errorcluster)  [unwired: 2 in, 2 out]
        n159 = invoke on="Conf In" class="Clust (strict)" method="Reinit To Default"(error in=w250) -> (error out=w270:errorcluster)  [unwired: 2 in, 2 out]
        n160 = invoke on="Current Sequence" class="Tbl (strict)" method="Reinit To Default"(error in=w250) -> (error out=w254:errorcluster)  [unwired: 2 in, 2 out]
        n161 = invoke on="Cond. Avan." class="Tbl (strict)" method="Reinit To Default"(error in=w250) -> (error out=w251:errorcluster)  [unwired: 2 in, 2 out]
        n162 = Merge Errors(w269, w270, w254, w251) -> (w268:errorcluster)
      }
      event "Open Cfg": Value Change {
        n163 = event-data() -> ()  [unwired: 1 in, 1 out]
        n164 = call <vilib>:"Application Directory.vi"() -> ("Application Directory"=w298:path)
        n165 = Build Path(base path=w298, name or relative path="Configuraciones") -> (appended path=w299:path)
        n166 = call "File Dialog"("start path"=w299, "pattern (all files)"="*.config", "pattern label"="Configuración SEC") -> ("selected path"=w294:path, "cancelled"=w301:bool, "error out"=w297:errorcluster)  [unwired: 9 in, 1 out]
        n167 = call <vilib>:"Clear Errors.vi"("error in (no error)"=w297) -> ()  [unwired: 5 in, 2 out]
        n168 = case shown="False" w301 {
          tunnel: w294 -> [w320 _]
          tunnel: w293 -> [w307 w336]
          tunnel: [w306 w336] -> w290
          tunnel: w292 -> [_ _]
          tunnel: w291 -> [w304 w335]
          tunnel: [w303 w335] -> w289
          tunnel: [w308 w334] -> w288
          tunnel: w287 -> [_ w334]
          frame False {
            n169 = Open/Create/Replace File(file path (use dialog)=w320, operation (0:open)=T20."open", access (0:read/write)=enum16{"read/write", "read-only", "write-only"}."read-only") -> (refnum out=w318:refnum<file>, error out=w316:errorcluster)  [unwired: 3 in, 1 out]
            n170 = Read from Binary File(5:"", 8:w316, 11:w318) -> (0:w315:errorcluster, 2:w313:string, 3:w317:refnum<file>)  [unwired: 3 in, 1 out]
            n171 = Bundle(w307) -> (w312:T23)  [unwired: 1 in]
            n172 = Unflatten From String(type=w312, binary string=w313) -> (value=w311:T23)  [unwired: 3 in, 2 out]
            n173 = Close File(refnum=w317, error in=w315) -> (error out=w314:errorcluster)  [unwired: 1 out]
            n174 = Unbundle(w311) -> (w306:T18)
            n175 = call <vilib>:"Clear Errors.vi"("error in (no error)"=w314) -> ()  [unwired: 5 in, 2 out]
            n176 = for {
              tunnel: w306 -> [w333] mode=indexing
              tunnel: [w324] -> w308 mode=indexing
              n177 = Unbundle By Name(w333) -> ("Progs Data"=w323:variant)
              n178 = Variant To Data(type=cluster{"I/O Map":T21, "Prog":T22} {"I/O Map"={"Inputs"=[], "Outputs"=[]}, "Prog"={"Prog. Data"={"Operación"=0, "Pieza"=0, "Descripción"="", "Nombre Programa"="", "Autor"="", "Diseño"="", "Total Meds.:"=0, "Total Meds. Aux.:"=0}, "All Sequences"={"Measurement"={"STEPs"=[], "Main Error&Alarm"={"Main Error"={"RPN "=[], "Variables"=[], "Ctes"=[], "Formula"="", "Message"=""}, "Main Alarm 1"={"RPN "=[], "Variables"=[], "Ctes"=[], "Formula"="", "Message"=""}, "Main Alarm 2"={"RPN "=[], "Variables"=[], "Ctes"=[], "Formula"="", "Message"=""}, "Main Alarm 3"={"RPN "=[], "Variables"=[], "Ctes"=[], "Formula"="", "Message"=""}, "Main Alarm 4"={"RPN "=[], "Variables"=[], "Ctes"=[], "Formula"="", "Message"=""}}}, "AutoZero"={"STEPs"=[], "Main Error&Alarm"={"Main Error"={"RPN "=[], "Variables"=[], "Ctes"=[], "Formula"="", "Message"=""}, "Main Alarm 1"={"RPN "=[], "Variables"=[], "Ctes"=[], "Formula"="", "Message"=""}, "Main Alarm 2"={"RPN "=[], "Variables"=[], "Ctes"=[], "Formula"="", "Message"=""}, "Main Alarm 3"={"RPN "=[], "Variables"=[], "Ctes"=[], "Formula"="", "Message"=""}, "Main Alarm 4"={"RPN "=[], "Variables"=[], "Ctes"=[], "Formula"="", "Message"=""}}}}}}, Variant=w323) -> (data=w325:cluster{"I/O Map":T21, "Prog":T22})  [unwired: 1 in, 1 out]
              n179 = Unbundle By Name(w325) -> ("Prog.Prog. Data.Nombre Programa"=w326:string, "Prog.Prog. Data.Descripción"=w327:string, "Prog.Prog. Data.Pieza"=w328:i32, "Prog.Prog. Data.Diseño"=w330:string, "Prog.Prog. Data.Operación"=w331:i32)
              n180 = Number To Decimal String(number=w328) -> (decimal integer string=w329:string)  [unwired: 1 in]
              n181 = Number To Decimal String(number=w331) -> (decimal integer string=w332:string)  [unwired: 1 in]
              n182 = Build Array("Arreglar" ("element"), w326, w327, w329, w330, w332) -> (w324:string[])
            }
            n183 = property on="Editor de Programas" class="MCListbox (strict)"(error in=w304, "Val(Sgnl)"=0 ("Value (Signaling)")) -> (error out=w303:errorcluster)  [unwired: 1 in, 1 out]
          }
          frame True {
          }
        }
      }
      event "Save Cfg": Value Change {
        n184 = event-data() -> ()  [unwired: 1 in, 6 out]
        n185 = call <vilib>:"Application Directory.vi"() -> ("Application Directory"=w346:path)
        n186 = Build Path(base path=w346, name or relative path="Configuraciones") -> (appended path=w348:path)
        n187 = Bundle(w340) -> (w349:T23)  [unwired: 1 in]
        n188 = call "File Dialog2"("start path"=w348, "pattern (all files)"="*.config", "pattern label"="Configuración SEC") -> ("selected path"=w341:path, "cancelled"=w344:bool, "error out"=w345:errorcluster)  [unwired: 9 in, 1 out]
        n189 = Flatten To String(anything=w349, error in (no error)=w338) -> (data string=w350:string, error out=w337:errorcluster)  [unwired: 2 in, 1 out]
        n190 = call <vilib>:"Clear Errors.vi"("error in (no error)"=w345) -> ()  [unwired: 5 in, 2 out]
        n191 = case shown="True" w344 {
          tunnel: w350 -> [w358 _]
          tunnel: w341 -> [w354 _]
          frame False {
            n192 = Open/Create/Replace File(file path (use dialog)=w354, operation (0:open)=T20."open or create", access (0:read/write)=enum16{"read/write", "read-only", "write-only"}."write-only") -> (refnum out=w355:refnum<file>, error out=w352:errorcluster)  [unwired: 3 in, 1 out]
            n193 = Write to Binary File(file (use dialog)=w355, data=w358, error in=w352) -> (refnum out=w353:refnum<file>, error out=w351:errorcluster)  [unwired: 3 in, 1 out]
            n194 = Close File(refnum=w353, error in=w351) -> ()  [unwired: 2 out]
          }
          frame True {
          }
        }
      }
      event "New Prog": Value Change {
        w366 = T13 {"File Direction"=path "", "Progs Data"=variant}  # Progs
        n195 = event-data() -> ()  [unwired: 1 in, 1 out]
        n196 = Matrix Size(0:w386) -> (1:w369:i32)  [unwired: 1 out]
        n197 = Number To Decimal String(number=w369) -> (decimal integer string=w377:string)  [unwired: 1 in]
        n198 = Index Array(array=w364, index=w363) -> (element=w359:T13)
        n199 = Concatenate Strings("Cod. Prog. ", w377) -> (w383:string)
        n200 = Concatenate Strings("Nombre Programa ", w377) -> (w382:string)
        n201 = Concatenate Strings("Descripción ", w377) -> (w381:string)
        n202 = Concatenate Strings("Pieza ", w377) -> (w380:string)
        n203 = Concatenate Strings("Diseño ", w377) -> (w379:string)
        n204 = Concatenate Strings("Operación ", w377) -> (w378:string)
        n205 = Build Array(w383, w382, w381, w380, w379, w378, "CAP" ("element")) -> (w384:string[])
        n206 = To Variant(anything=w359) -> (Variant=w365:variant)
        n207 = call-poly "Enqueue Message.vi"("error in (no error)"=w360, "Message Data"=w365, "Message"="INIT", "Message Queue"=w362) -> ("error out"=w367:errorcluster)  [unwired: 6 in, 1 out]
        n208 = Insert Into Array(array=w364, index=w369, new element=w366) -> (w370:T18)
        n209 = Insert Into Array(array=w386, index (row)=w369, new element=w384) -> (w387:string[][])  [unwired: 1 in]
        n210 = property on="Editor de Programas" class="MCListbox (strict)"(error in=w367, "Value"=w369) -> (error out=w385:errorcluster)  [unwired: 1 in, 1 out]
      }
      event "HOME": Value Change {
        n211 = event-data() -> ()  [unwired: 1 in, 1 out]
        n212 = property on="Tab Control 2" class="TabCtl (strict)"(error in=w390, "Value"=enum32{"HOME", "PIC", "TAB"}."HOME" ("Tab Control 2")) -> (error out=w394:errorcluster)  [unwired: 1 in, 1 out]
        n213 = property on="Tab Control" class="TabCtl (strict)"(error in=w390, "Value"=enum32{"HOME", "SEC", "MIMIC", "MESSAGE"}."HOME" ("Tab Control")) -> (error out=w408:errorcluster)  [unwired: 1 in, 1 out]
        n214 = property on="SEC" class="Bool (strict)"(error in=w390, "Value"=FALSE ("CICLO")) -> (error out=w410:errorcluster)  [unwired: 1 in, 1 out]
        n215 = property on="MIMIC" class="Bool (strict)"(error in=w390, "Value"=FALSE ("CONFIG.")) -> (error out=w397:errorcluster)  [unwired: 1 in, 1 out]
        n216 = property on="MESSAGE" class="Bool (strict)"(error in=w390, "Value"=FALSE ("CONFIG.")) -> (error out=w388:errorcluster)  [unwired: 1 in, 1 out]
        n217 = property on="MESSAGE" class="Bool (strict)"(error in=w390, "DisabledEnum"=T11."Enabled" ("Disabled")) -> (error out=w393:errorcluster)  [unwired: 1 in, 1 out]
        n218 = property on="SEC" class="Bool (strict)"(error in=w390, "DisabledEnum"=T11."Enabled" ("Disabled")) -> (error out=w398:errorcluster)  [unwired: 1 in, 1 out]
        n219 = property on="MIMIC" class="Bool (strict)"(error in=w390, "DisabledEnum"=T11."Enabled" ("Disabled")) -> (error out=w399:errorcluster)  [unwired: 1 in, 1 out]
        n220 = property on="HOME" class="Bool (strict)"(error in=w390, "DisabledEnum"=T11."Disabled" ("Disabled")) -> (error out=w389:errorcluster)  [unwired: 1 in, 1 out]
        n221 = Merge Errors(w394, w393, w398, w399, w408, w410, w397, w388, w389) -> (w406:errorcluster)
      }
      event "SEC": Value Change {
        w411 = T3 {"Boolean 36"=FALSE, "Boolean 3"=FALSE, "Boolean 35"=FALSE, "Boolean 34"=FALSE, "Boolean 33"=FALSE, "Boolean 32"=FALSE, "Boolean 16"=FALSE, "Boolean 17"=FALSE, "Boolean 26"=FALSE, "Boolean 25"=FALSE, "Boolean 24"=FALSE, "Boolean 23"=FALSE, "Boolean 37"=FALSE, "Boolean 1"=FALSE, "Boolean 15"=FALSE, "Boolean 4"=FALSE, "Boolean 5"=FALSE, "Boolean 6"=FALSE, "Boolean 7"=FALSE, "Boolean 8"=FALSE, "Boolean 9"=FALSE, "Boolean 10"=FALSE, "Boolean 11"=FALSE, "Boolean 12"=FALSE, "Boolean 38"=FALSE, "Boolean 21"=FALSE, "Boolean 22"=FALSE, "Boolean 20"=FALSE, "Boolean 19"=FALSE, "Boolean 18"=FALSE, "Boolean 40"=FALSE, "Boolean 39"=FALSE} ("View Out")
        n222 = event-data() -> ()  [unwired: 1 in, 1 out]
        n223 = property on="Tab Control 2" class="TabCtl (strict)"(error in=w412, "Value"=enum32{"HOME", "PIC", "TAB"}."PIC" ("Tab Control 2")) -> (error out=w423:errorcluster)  [unwired: 1 in, 1 out]
        n224 = property on="Tab Control" class="TabCtl (strict)"(error in=w412, "Value"=enum32{"HOME", "SEC", "MIMIC", "MESSAGE"}."SEC" ("Tab Control")) -> (error out=w432:errorcluster)  [unwired: 1 in, 1 out]
        n225 = property on="MESSAGE" class="Bool (strict)"(error in=w412, "Value"=FALSE ("CICLO")) -> (error out=w415:errorcluster)  [unwired: 1 in, 1 out]
        n226 = property on="HOME" class="Bool (strict)"(error in=w412, "Value"=FALSE ("CICLO")) -> (error out=w416:errorcluster)  [unwired: 1 in, 1 out]
        n227 = property on="MIMIC" class="Bool (strict)"(error in=w412, "Value"=FALSE ("CONFIG.")) -> (error out=w417:errorcluster)  [unwired: 1 in, 1 out]
        n228 = property on="HOME" class="Bool (strict)"(error in=w412, "DisabledEnum"=T11."Enabled" ("Disabled")) -> (error out=w422:errorcluster)  [unwired: 1 in, 1 out]
        n229 = property on="MIMIC" class="Bool (strict)"(error in=w412, "DisabledEnum"=T11."Enabled" ("Disabled")) -> (error out=w421:errorcluster)  [unwired: 1 in, 1 out]
        n230 = property on="MESSAGE" class="Bool (strict)"(error in=w412, "DisabledEnum"=T11."Enabled" ("Disabled")) -> (error out=w420:errorcluster)  [unwired: 1 in, 1 out]
        n231 = property on="SEC" class="Bool (strict)"(error in=w412, "DisabledEnum"=T11."Disabled" ("Disabled")) -> (error out=w418:errorcluster)  [unwired: 1 in, 1 out]
        n232 = Merge Errors(w423, w422, w421, w420, w432, w415, w416, w417, w418) -> (w434:errorcluster)
        n233 = global write "DO Monitoring Global Variables.vi" "View Out"(w411) -> ()
        n234 = global write "DO Monitoring Global Variables.vi" "View Out 2"(w411) -> ()
        n235 = global write "DO Monitoring Global Variables.vi" "View Out 3"(w411) -> ()
        n236 = global write "DO Monitoring Global Variables.vi" "View Out 4"(w411) -> ()
        n237 = global write "DO Monitoring Global Variables.vi" "View Out 5"(w411) -> ()
      }
      event "MIMIC": Value Change {
        n238 = event-data() -> ()  [unwired: 1 in, 1 out]
        n239 = property on="Tab Control 2" class="TabCtl (strict)"(error in=w435, "Value"=enum32{"HOME", "PIC", "TAB"}."TAB" ("Tab Control 2")) -> (error out=w440:errorcluster)  [unwired: 1 in, 1 out]
        n240 = property on="Tab Control" class="TabCtl (strict)"(error in=w435, "Value"=enum32{"HOME", "SEC", "MIMIC", "MESSAGE"}."MIMIC" ("Tab Control")) -> (error out=w455:errorcluster)  [unwired: 1 in, 1 out]
        n241 = property on="HOME" class="Bool (strict)"(error in=w435, "Value"=FALSE ("CICLO")) -> (error out=w457:errorcluster)  [unwired: 1 in, 1 out]
        n242 = property on="SEC" class="Bool (strict)"(error in=w435, "Value"=FALSE ("CONFIG.")) -> (error out=w445:errorcluster)  [unwired: 1 in, 1 out]
        n243 = property on="MESSAGE" class="Bool (strict)"(error in=w435, "Value"=FALSE ("CONFIG.")) -> (error out=w436:errorcluster)  [unwired: 1 in, 1 out]
        n244 = property on="MESSAGE" class="Bool (strict)"(error in=w435, "DisabledEnum"=T11."Enabled" ("Disabled")) -> (error out=w439:errorcluster)  [unwired: 1 in, 1 out]
        n245 = property on="HOME" class="Bool (strict)"(error in=w435, "DisabledEnum"=T11."Enabled" ("Disabled")) -> (error out=w446:errorcluster)  [unwired: 1 in, 1 out]
        n246 = property on="SEC" class="Bool (strict)"(error in=w435, "DisabledEnum"=T11."Enabled" ("Disabled")) -> (error out=w447:errorcluster)  [unwired: 1 in, 1 out]
        n247 = property on="MIMIC" class="Bool (strict)"(error in=w435, "DisabledEnum"=T11."Disabled" ("Disabled")) -> (error out=w437:errorcluster)  [unwired: 1 in, 1 out]
        n248 = Merge Errors(w440, w439, w446, w447, w455, w457, w445, w436, w437) -> (w454:errorcluster)
      }
      event "MESSAGE": Value Change {
        n249 = event-data() -> ()  [unwired: 1 in, 1 out]
        n250 = property on="Tab Control 2" class="TabCtl (strict)"(error in=w460, "Value"=enum32{"HOME", "PIC", "TAB"}."TAB" ("Tab Control 2")) -> (error out=w463:errorcluster)  [unwired: 1 in, 1 out]
        n251 = property on="Tab Control" class="TabCtl (strict)"(error in=w460, "Value"=enum32{"HOME", "SEC", "MIMIC", "MESSAGE"}."MESSAGE" ("Tab Control")) -> (error out=w475:errorcluster)  [unwired: 1 in, 1 out]
        n252 = property on="HOME" class="Bool (strict)"(error in=w460, "Value"=FALSE ("CICLO")) -> (error out=w477:errorcluster)  [unwired: 1 in, 1 out]
        n253 = property on="SEC" class="Bool (strict)"(error in=w460, "Value"=FALSE ("CONFIG.")) -> (error out=w469:errorcluster)  [unwired: 1 in, 1 out]
        n254 = property on="MIMIC" class="Bool (strict)"(error in=w460, "Value"=FALSE ("CONFIG.")) -> (error out=w458:errorcluster)  [unwired: 1 in, 1 out]
        n255 = property on="MIMIC" class="Bool (strict)"(error in=w460, "DisabledEnum"=T11."Enabled" ("Disabled")) -> (error out=w462:errorcluster)  [unwired: 1 in, 1 out]
        n256 = property on="HOME" class="Bool (strict)"(error in=w460, "DisabledEnum"=T11."Enabled" ("Disabled")) -> (error out=w470:errorcluster)  [unwired: 1 in, 1 out]
        n257 = property on="SEC" class="Bool (strict)"(error in=w460, "DisabledEnum"=T11."Enabled" ("Disabled")) -> (error out=w471:errorcluster)  [unwired: 1 in, 1 out]
        n258 = property on="MESSAGE" class="Bool (strict)"(error in=w460, "DisabledEnum"=T11."Disabled" ("Disabled")) -> (error out=w459:errorcluster)  [unwired: 1 in, 1 out]
        n259 = Merge Errors(w463, w462, w470, w471, w475, w477, w469, w458, w459) -> (w467:errorcluster)
      }
      event "I/O Config": Value Change {
        n260 = event-data() -> ()  [unwired: 1 in, 1 out]
        n261 = call-poly "Enqueue Message.vi"("error in (no error)"=w482, "Message"="Config:IO", "Message Queue"=w483) -> ("error out"=w481:errorcluster, "dup Message Queue"=w486:refnum<queue>)  [unwired: 7 in]
        n262 = call-poly "Enqueue Message.vi"("error in (no error)"=w481, "Message"="Config:Get", "Message Queue"=w486) -> ("error out"=w480:errorcluster)  [unwired: 7 in, 1 out]
      }
      event "Config Prog": Value Change {
        n263 = event-data() -> ()  [unwired: 1 in, 1 out]
        n264 = Index Array(array=w494, index (row)=w493, index (col)=6 ("disabled index (col)")) -> (element=w491:string)
        n265 = To Variant(anything=w491) -> (Variant=w490:variant)
        n266 = call-poly "Enqueue Message.vi"("error in (no error)"=w497, "Message Data"=w490, "Message"="Config", "Message Queue"=w496) -> ("error out"=w498:errorcluster, "dup Message Queue"=w499:refnum<queue>)  [unwired: 6 in]
        n267 = call-poly "Enqueue Message.vi"("Message"="Config:Get", "Message Queue"=w499) -> ()  [unwired: 8 in, 2 out]
      }
      event User Event {
        n268 = event-data() -> ("Config Data"=w505:variant)  [unwired: 1 in]
        n269 = in-place {
          in-place-border: w505 -> [w521]
          n270 = in-place-array #4(w520, w513) -> (w523:T13)
          n271 = Bundle By Name(cluster=w523, "Progs Data"=w521) -> (w522:T13)
          n272 = in-place-array #4(w522) -> (w519:T18)  [unwired: 1 out]
        }
        n273 = Variant To Data(error in=w504, type=cluster{"I/O Map":T21, "Prog":T22} {"I/O Map"={"Inputs"=[], "Outputs"=[]}, "Prog"={"Prog. Data"={"Operación"=0, "Pieza"=0, "Descripción"="", "Nombre Programa"="", "Autor"="", "Diseño"="", "Total Meds.:"=0, "Total Meds. Aux.:"=0}, "All Sequences"={"Measurement"={"STEPs"=[], "Main Error&Alarm"={"Main Error"={"RPN "=[], "Variables"=[], "Ctes"=[], "Formula"="", "Message"=""}, "Main Alarm 1"={"RPN "=[], "Variables"=[], "Ctes"=[], "Formula"="", "Message"=""}, "Main Alarm 2"={"RPN "=[], "Variables"=[], "Ctes"=[], "Formula"="", "Message"=""}, "Main Alarm 3"={"RPN "=[], "Variables"=[], "Ctes"=[], "Formula"="", "Message"=""}, "Main Alarm 4"={"RPN "=[], "Variables"=[], "Ctes"=[], "Formula"="", "Message"=""}}}, "AutoZero"={"STEPs"=[], "Main Error&Alarm"={"Main Error"={"RPN "=[], "Variables"=[], "Ctes"=[], "Formula"="", "Message"=""}, "Main Alarm 1"={"RPN "=[], "Variables"=[], "Ctes"=[], "Formula"="", "Message"=""}, "Main Alarm 2"={"RPN "=[], "Variables"=[], "Ctes"=[], "Formula"="", "Message"=""}, "Main Alarm 3"={"RPN "=[], "Variables"=[], "Ctes"=[], "Formula"="", "Message"=""}, "Main Alarm 4"={"RPN "=[], "Variables"=[], "Ctes"=[], "Formula"="", "Message"=""}}}}}}, Variant=w505) -> (data=w517:cluster{"I/O Map":T21, "Prog":T22}, error out=w518:errorcluster)
        n274 = Unbundle By Name(w517) -> ("Prog.Prog. Data.Nombre Programa"=w512:string, "Prog.Prog. Data.Descripción"=w511:string, "Prog.Prog. Data.Pieza"=w510:i32, "Prog.Prog. Data.Diseño"=w508:string, "Prog.Prog. Data.Operación"=w507:i32)
        n275 = Number To Decimal String(number=w510) -> (decimal integer string=w509:string)  [unwired: 1 in]
        n276 = Number To Decimal String(number=w507) -> (decimal integer string=w506:string)  [unwired: 1 in]
        n277 = Build Array("arreglar" ("element"), w512, w511, w509, w508, w506) -> (w514:string[])
        n278 = Replace Array Subset(array=w516, new element=w514, index (row)=w513) -> (w515:string[][])  [unwired: 1 in]
      }
      event "Start Sec A-Z": Value Change {
        w524 = T3 {"Boolean 36"=FALSE, "Boolean 3"=FALSE, "Boolean 35"=FALSE, "Boolean 34"=FALSE, "Boolean 33"=FALSE, "Boolean 32"=FALSE, "Boolean 16"=FALSE, "Boolean 17"=FALSE, "Boolean 26"=FALSE, "Boolean 25"=FALSE, "Boolean 24"=FALSE, "Boolean 23"=FALSE, "Boolean 37"=FALSE, "Boolean 1"=FALSE, "Boolean 15"=FALSE, "Boolean 4"=FALSE, "Boolean 5"=FALSE, "Boolean 6"=FALSE, "Boolean 7"=FALSE, "Boolean 8"=FALSE, "Boolean 9"=FALSE, "Boolean 10"=FALSE, "Boolean 11"=FALSE, "Boolean 12"=FALSE, "Boolean 38"=FALSE, "Boolean 21"=FALSE, "Boolean 22"=FALSE, "Boolean 20"=FALSE, "Boolean 19"=FALSE, "Boolean 18"=FALSE, "Boolean 40"=FALSE, "Boolean 39"=FALSE} ("View Out")
        w531 = T14 {"Row"=-2, "Column"=-2} ("Active Cell:Active Cell")
        w534 = T14 {"Row"=0, "Column"=-2} ("Active Cell:Active Cell")
        w535 = u32 4110335
        w532 = u32 16448250
        n279 = event-data() -> ()  [unwired: 1 in, 1 out]
        n280 = To Variant(anything="Auto-Zero") -> (Variant=w537:variant)
        n281 = call-poly "Enqueue Message.vi"("error in (no error)"=w527, "Message Data"=w537, "Message"="Start", "Message Queue"=w544) -> ("error out"=w533:errorcluster)  [unwired: 6 in, 1 out]
        n282 = call-poly "Enqueue Message.vi"("error in (no error)"=w527, "Message"="Init", "Message Queue"=w526) -> ()  [unwired: 7 in, 2 out]
        n283 = property on="Cond. Avan." class="Tbl (strict)"(error in=w533, "Active Cell"=w531, "Cell BG Color"=w532) -> (error out=w536:errorcluster)  [unwired: 1 in, 1 out]
        n284 = property on="Current Sequence" class="Tbl (strict)"(error in=w533, "Active Cell"=w531, "Cell BG Color"=w532) -> (error out=w539:errorcluster)  [unwired: 1 in, 1 out]
        n285 = global write "DO Monitoring Global Variables.vi" "View Out"(w524) -> ()
        n286 = global write "DO Monitoring Global Variables.vi" "View Out 2"(w524) -> ()
        n287 = global write "DO Monitoring Global Variables.vi" "View Out 3"(w524) -> ()
        n288 = global write "DO Monitoring Global Variables.vi" "View Out 4"(w524) -> ()
        n289 = global write "DO Monitoring Global Variables.vi" "View Out 5"(w524) -> ()
        n290 = property on="Cond. Avan." class="Tbl (strict)"(error in=w536, "Active Cell"=w534, "Cell BG Color"=w535) -> (error out=w530:errorcluster)  [unwired: 1 in, 1 out]
        n291 = property on="Current Sequence" class="Tbl (strict)"(error in=w539, "Active Cell"=w534, "Cell BG Color"=w535) -> (error out=w529:errorcluster)  [unwired: 1 in, 1 out]
        n292 = Merge Errors(w530, w529) -> (w525:errorcluster)
      }
      event "Start Sec Ciclo": Value Change {
        w545 = T3 {"Boolean 36"=FALSE, "Boolean 3"=FALSE, "Boolean 35"=FALSE, "Boolean 34"=FALSE, "Boolean 33"=FALSE, "Boolean 32"=FALSE, "Boolean 16"=FALSE, "Boolean 17"=FALSE, "Boolean 26"=FALSE, "Boolean 25"=FALSE, "Boolean 24"=FALSE, "Boolean 23"=FALSE, "Boolean 37"=FALSE, "Boolean 1"=FALSE, "Boolean 15"=FALSE, "Boolean 4"=FALSE, "Boolean 5"=FALSE, "Boolean 6"=FALSE, "Boolean 7"=FALSE, "Boolean 8"=FALSE, "Boolean 9"=FALSE, "Boolean 10"=FALSE, "Boolean 11"=FALSE, "Boolean 12"=FALSE, "Boolean 38"=FALSE, "Boolean 21"=FALSE, "Boolean 22"=FALSE, "Boolean 20"=FALSE, "Boolean 19"=FALSE, "Boolean 18"=FALSE, "Boolean 40"=FALSE, "Boolean 39"=FALSE} ("View Out")
        w552 = T14 {"Row"=0, "Column"=-2} ("Active Cell:Active Cell")
        w553 = u32 4110335
        w555 = T14 {"Row"=-2, "Column"=-2} ("Active Cell:Active Cell")
        w554 = u32 16448250
        n293 = event-data() -> ()  [unwired: 1 in, 1 out]
        n294 = To Variant(anything="Measurement") -> (Variant=w558:variant)
        n295 = call-poly "Enqueue Message.vi"("error in (no error)"=w548, "Message"="Init", "Message Queue"=w547) -> ()  [unwired: 7 in, 2 out]
        n296 = call-poly "Enqueue Message.vi"("error in (no error)"=w548, "Message Data"=w558, "Message"="Start", "Message Queue"=w564) -> ("error out"=w556:errorcluster)  [unwired: 6 in, 1 out]
        n297 = property on="Cond. Avan." class="Tbl (strict)"(error in=w556, "Active Cell"=w555, "Cell BG Color"=w554) -> (error out=w557:errorcluster)  [unwired: 1 in, 1 out]
        n298 = property on="Current Sequence" class="Tbl (strict)"(error in=w556, "Active Cell"=w555, "Cell BG Color"=w554) -> (error out=w560:errorcluster)  [unwired: 1 in, 1 out]
        n299 = property on="Cond. Avan." class="Tbl (strict)"(error in=w557, "Active Cell"=w552, "Cell BG Color"=w553) -> (error out=w551:errorcluster)  [unwired: 1 in, 1 out]
        n300 = property on="Current Sequence" class="Tbl (strict)"(error in=w560, "Active Cell"=w552, "Cell BG Color"=w553) -> (error out=w550:errorcluster)  [unwired: 1 in, 1 out]
        n301 = Merge Errors(w551, w550) -> (w546:errorcluster)
        n302 = global write "DO Monitoring Global Variables.vi" "View Out"(w545) -> ()
        n303 = global write "DO Monitoring Global Variables.vi" "View Out 2"(w545) -> ()
        n304 = global write "DO Monitoring Global Variables.vi" "View Out 3"(w545) -> ()
        n305 = global write "DO Monitoring Global Variables.vi" "View Out 4"(w545) -> ()
        n306 = global write "DO Monitoring Global Variables.vi" "View Out 5"(w545) -> ()
      }
      event "Acept": Value Change {
        n307 = event-data() -> ()  [unwired: 1 in, 1 out]
        n308 = flat-sequence {
          tunnel: [w573] -> w570
          tunnel: w569 -> [w573]
          tunnel: w570 -> [w576]
          tunnel: [w575] -> w568
          tunnel: w568 -> [w595]
          tunnel: [w594] -> w567
          frame #0 {
            n309 = local write "Acept"(FALSE ("Acept")) -> ()
          }
          frame #1 {
            n310 = for {
              N: 13 -> [_]
              shift-right: [w584] -> _
              shift-left: "" ("Boolean Text.Text") -> [w589]
              tunnel: w576 -> [w581]
              tunnel: [w580] -> w575
              i -> [w593]
              n311 = Equal?(x=0, y=w593) -> (x = y?=w591:bool)
              n312 = Select(t="CONTROLANDO" ("Boolean Text.Text"), s=w591, f=". " ("Boolean Text.Text")) -> (s? t:f=w588:string)
              n313 = Concatenate Strings(w589, w588) -> (w585:string)
              n314 = Equal?(x="CONTROLANDO. . . " ("Boolean Text.Text"), y=w585) -> (x = y?=w586:bool)
              n315 = property on="Acept" class="Bool"(error in=w581, "BoolText.Text"=w585) -> (error out=w580:errorcluster)  [unwired: 1 in, 1 out]
              n316 = Select(t="CONTROLANDO" ("Boolean Text.Text"), s=w586, f=w585) -> (s? t:f=w584:string)
              n317 = Wait (ms)(milliseconds to wait=u32 200) -> ()  [unwired: 1 out]
            }
          }
          frame #2 {
            n318 = property on="Acept" class="Bool"(error in=w595, "BoolText.Text"="       ACEPTADO" ("Boolean Text.Text")) -> (error out=w594:errorcluster)  [unwired: 1 in, 1 out]
            "Acept" <- TRUE ("Acept")
          }
        }
      }
      event "Conf In", "Conf In 2", "Conf In 3", "Conf In 4", "Conf In 5", "Angle": Value Change {
        w615 = T24 {"Encoder"=0.0, "DI"=[], "DO"=[]} ("Control Data")
        n319 = event-data() -> ()  [unwired: 1 in, 1 out]
        n320 = Unbundle By Name(w603) -> ("CTRL HWSync1"=w598:refnum<notifier>, "CTRL HWSync2"=w599:refnum<notifier>, "CTRL HWSync3"=w600:refnum<notifier>, "CTRL HWSync4"=w601:refnum<notifier>, "CTRL HWSync5"=w602:refnum<notifier>)
        n321 = Cluster To Array(cluster="Conf In") -> (array=w624:bool[])
        n322 = Cluster To Array(cluster="Conf In 2") -> (array=w623:bool[])
        n323 = Cluster To Array(cluster="Conf In 3") -> (array=w617:bool[])
        n324 = Cluster To Array(cluster="Conf In 4") -> (array=w616:bool[])
        n325 = Cluster To Array(cluster="Conf In 5") -> (array=w620:bool[])
        n326 = Bundle By Name(cluster=w615, "DI"=w624, "Encoder"="Angle") -> (w627:T24)
        n327 = Bundle By Name(cluster=w615, "DI"=w623) -> (w621:T24)
        n328 = Bundle By Name(cluster=w615, "DI"=w617) -> (w612:T24)
        n329 = Bundle By Name(cluster=w615, "DI"=w616) -> (w611:T24)
        n330 = Bundle By Name(cluster=w615, "DI"=w620) -> (w618:T24)
        n331 = call "Send CTRL Notification.vi"("error in (no error)"=w610, "Control Data"=w627, "CTRL Data Notifier in"=w598) -> ("error out"=w609:errorcluster)  [unwired: 7 in, 1 out]
        n332 = call "Send CTRL Notification.vi"("error in (no error)"=w610, "Control Data"=w621, "CTRL Data Notifier in"=w599) -> ("error out"=w608:errorcluster)  [unwired: 7 in, 1 out]
        n333 = call "Send CTRL Notification.vi"("error in (no error)"=w610, "Control Data"=w612, "CTRL Data Notifier in"=w600) -> ("error out"=w607:errorcluster)  [unwired: 7 in, 1 out]
        n334 = call "Send CTRL Notification.vi"("error in (no error)"=w610, "Control Data"=w611, "CTRL Data Notifier in"=w601) -> ("error out"=w606:errorcluster)  [unwired: 7 in, 1 out]
        n335 = call "Send CTRL Notification.vi"("error in (no error)"=w610, "Control Data"=w618, "CTRL Data Notifier in"=w602) -> ("error out"=w605:errorcluster)  [unwired: 7 in, 1 out]
        n336 = Merge Errors(w609, w608, w607, w606, w605) -> (w604:errorcluster)
      }
      event Panel Close? {
        n337 = event-data() -> ()  [unwired: 1 in, 1 out]
        n338 = call-poly "Enqueue Message.vi"("error in (no error)"=w638, "Message"="EXIT", "Message Queue"=w634) -> ("error out"=w637:errorcluster)  [unwired: 7 in, 1 out]
        n339 = call-poly "Enqueue Message.vi"("error in (no error)"=w637, "Message"="EXIT", "Message Queue"=w635) -> ("error out"=w636:errorcluster)  [unwired: 7 in, 1 out]
        n340 = event-data("Discard?"=TRUE) -> ()  [unwired: 1 in, 1 out]
      }
    }
    n341 = property on="Editor de Programas" class="MCListbox (strict)"(error in=w193, "ItemNames"=w187) -> ()  [unwired: 1 in, 2 out]
  }
  n342 = while {
    tunnel: [w651] -> _
    tunnel: w97 -> [w647]
    tunnel: w56 -> [w646]
    tunnel: w94 -> [w645]
    shift-right: [w643] -> _
    shift-left: T10 {"HWS1"="", "HWS2"="", "HWS3"="", "HWS4"="", "HWS5"="", "MATH"=""} -> [w644]
    stop <- w652 stop-if-true
    # "HAL Message Switch Loop"
    n343 = call "Dequeue Message.vi"("error in (no error)"=w646, "Message Queue"=w647) -> ("error out"=w650:errorcluster, "Message Data"=w649:variant, "Message"=w648:string)  [unwired: 6 in, 1 out]
    n344 = case shown="\"EXIT\"" w648 {
      selector: w648 -> [w659 _ _ _]
      tunnel: w650 -> [w663 w888 w891 w917]
      tunnel: w649 -> [w658 _ _ w919]
      tunnel: [_ TRUE _ _] -> w652
      tunnel: [w663 w888 w890 w916] -> w651
      tunnel: w645 -> [_ _ _ w918]
      tunnel: w644 -> [w656 w887 _ w915]
      tunnel: [w657 w887 T10 {"HWS1"="", "HWS2"="", "HWS3"="", "HWS4"="", "HWS5"="", "MATH"=""} w915] -> w643
      frame Default {
        n345 = Get Date/Time In Seconds() -> (seconds since 1Jan1904=w654:timestamp)
        n346 = Match Pattern(string=w659, regular expression=":") -> (before substring=w661:string, after substring=w660:string)  [unwired: 1 in, 2 out]
        n347 = Format Date/Time String(time format string (%c)="%H:%M:%S%3u ", seconds (now)=w654) -> (date/time string=w653:string)  [unwired: 1 in]
        n348 = case shown="\"MATH\"" w661 {
          tunnel: w660 -> [_ w671 w791]
          tunnel: w658 -> [_ w668 w792]
          tunnel: w656 -> [w664 w667 w788]
          tunnel: [w664 w666 w789] -> w657
          tunnel: w653 -> [_ w665 w790]
          frame Default {
          }
          frame "HAL" {
            n349 = Match Pattern(string=w671, regular expression=":") -> (before substring=w670:string, after substring=w669:string)  [unwired: 1 in, 2 out]
            n350 = case shown="\"HWSync1\"" w670 {
              tunnel: w669 -> [_ w675 w689 w705 w717 w731 w746 w750 w754 w758 w762 w766 w770 w774 w778 w782]
              tunnel: w668 -> [_ w682 w695 w710 w724 w738 _ _ _ _ _ _ _ _ _ _]
              tunnel: w667 -> [w673 w681 w693 w708 w721 w737 w744 w748 w752 w756 w760 w764 w768 w772 w776 w780]
              tunnel: [w673 w680 w694 w707 w722 w736 w744 w748 w752 w756 w760 w764 w768 w772 w776 w780] -> w666
              tunnel: w665 -> [_ w674 w688 w702 w716 w730 _ _ _ _ _ _ _ _ _ _]
              frame "False", Default {
              }
              frame "HWSync1" {
                n351 = Unbundle By Name(w681) -> ("HWS1"=w676:string)
                n352 = Match Pattern(string=w675, regular expression=":") -> (before substring=w678:string)  [unwired: 1 in, 3 out]
                n353 = case shown="\"Digital Out Write\"" w678 {
                  tunnel: w682 -> [_ w687]
                  frame "False", Default {
                  }
                  frame "Digital Out Write" {
                    n354 = Variant To Data(type=0, Variant=w687) -> (data=w685:i32)  [unwired: 1 in, 1 out]
                    n355 = Number To Boolean Array(number=w685) -> (Boolean array=→"DO 1":bool[])
                  }
                }
                n356 = Concatenate Strings(w676, w674, w675, "\r\n") -> (w679:string)
                "HWSync 1" <- w679
                n357 = Bundle By Name(cluster=w681, "HWS1"=w679) -> (w680:T10)
              }
              frame "HWSync2" {
                n358 = Unbundle By Name(w693) -> ("HWS2"=w691:string)
                n359 = Match Pattern(string=w689, regular expression=":") -> (before substring=w696:string)  [unwired: 1 in, 3 out]
                n360 = case shown="\"Digital Out Write\"" w696 {
                  tunnel: w695 -> [_ w701]
                  frame "False", Default {
                  }
                  frame "Digital Out Write" {
                    n361 = Variant To Data(type=0, Variant=w701) -> (data=w699:i32)  [unwired: 1 in, 1 out]
                    n362 = Number To Boolean Array(number=w699) -> (Boolean array=→"DO 2":bool[])
                  }
                }
                n363 = Concatenate Strings(w691, w688, w689, "\r\n") -> (w690:string)
                "HWSync 2" <- w690
                n364 = Bundle By Name(cluster=w693, "HWS2"=w690) -> (w694:T10)
              }
              frame "HWSync3" {
                n365 = Unbundle By Name(w708) -> ("HWS3"=w704:string)
                n366 = Match Pattern(string=w705, regular expression=":") -> (before substring=w709:string)  [unwired: 1 in, 3 out]
                n367 = case shown="\"Digital Out Write\"" w709 {
                  tunnel: w710 -> [_ w715]
                  frame "False", Default {
                  }
                  frame "Digital Out Write" {
                    n368 = Variant To Data(type=0, Variant=w715) -> (data=w713:i32)  [unwired: 1 in, 1 out]
                    n369 = Number To Boolean Array(number=w713) -> (Boolean array=→"DO 3":bool[])
                  }
                }
                n370 = Concatenate Strings(w704, w702, w705, "\r\n") -> (w703:string)
                "HWSync 3" <- w703
                n371 = Bundle By Name(cluster=w708, "HWS3"=w703) -> (w707:T10)
              }
              frame "HWSync4" {
                n372 = Unbundle By Name(w721) -> ("HWS4"=w719:string)
                n373 = Match Pattern(string=w717, regular expression=":") -> (before substring=w723:string)  [unwired: 1 in, 3 out]
                n374 = case shown="\"Digital Out Write\"" w723 {
                  tunnel: w724 -> [_ w729]
                  frame "False", Default {
                  }
                  frame "Digital Out Write" {
                    n375 = Variant To Data(type=0, Variant=w729) -> (data=w727:i32)  [unwired: 1 in, 1 out]
                    n376 = Number To Boolean Array(number=w727) -> (Boolean array=→"DO 4":bool[])
                  }
                }
                n377 = Concatenate Strings(w719, w716, w717, "\r\n") -> (w718:string)
                "HWSync 4" <- w718
                n378 = Bundle By Name(cluster=w721, "HWS4"=w718) -> (w722:T10)
              }
              frame "HWSync5" {
                n379 = Unbundle By Name(w737) -> ("HWS5"=w733:string)
                n380 = Match Pattern(string=w731, regular expression=":") -> (before substring=w735:string)  [unwired: 1 in, 3 out]
                n381 = case shown="\"Digital Out Write\"" w735 {
                  tunnel: w738 -> [_ w743]
                  frame "False", Default {
                  }
                  frame "Digital Out Write" {
                    n382 = Variant To Data(type=0, Variant=w743) -> (data=w741:i32)  [unwired: 1 in, 1 out]
                    n383 = Number To Boolean Array(number=w741) -> (Boolean array=→"DO 5":bool[])
                  }
                }
                n384 = Concatenate Strings(w733, w730, w731, "\r\n") -> (w732:string)
                "HWSync 5" <- w732
                n385 = Bundle By Name(cluster=w737, "HWS5"=w732) -> (w736:T10)
              }
              frame "HWAsync1" {
                n386 = Match Pattern(string=w746, regular expression=":") -> (before substring=→"HWAsync 1":string)  [unwired: 1 in, 3 out]
              }
              frame "HWAsync2" {
                n387 = Match Pattern(string=w750, regular expression=":") -> (before substring=→"HWAsync 2":string)  [unwired: 1 in, 3 out]
              }
              frame "HWAsync3" {
                n388 = Match Pattern(string=w754, regular expression=":") -> (before substring=→"HWAsync 3":string)  [unwired: 1 in, 3 out]
              }
              frame "HWAsync4" {
                n389 = Match Pattern(string=w758, regular expression=":") -> (before substring=→"HWAsync 4":string)  [unwired: 1 in, 3 out]
              }
              frame "HWAsync5" {
                n390 = Match Pattern(string=w762, regular expression=":") -> (before substring=→"HWAsync 5":string)  [unwired: 1 in, 3 out]
              }
              frame "HWAsync6" {
                n391 = Match Pattern(string=w766, regular expression=":") -> (before substring=→"HWAsync 6":string)  [unwired: 1 in, 3 out]
              }
              frame "HWAsync7" {
                n392 = Match Pattern(string=w770, regular expression=":") -> (before substring=→"HWAsync 7":string)  [unwired: 1 in, 3 out]
              }
              frame "HWAsync8" {
                n393 = Match Pattern(string=w774, regular expression=":") -> (before substring=→"HWAsync 8":string)  [unwired: 1 in, 3 out]
              }
              frame "HWAsync9" {
                n394 = Match Pattern(string=w778, regular expression=":") -> (before substring=→"HWAsync 9":string)  [unwired: 1 in, 3 out]
              }
              frame "HWAsync10" {
                n395 = Match Pattern(string=w782, regular expression=":") -> (before substring=→"HWAsync 10":string)  [unwired: 1 in, 3 out]
              }
            }
          }
          frame "MATH" {
            n396 = case shown="Default" w791 {
              tunnel: w792 -> [_ w800 w856 w871 w883 _]
              tunnel: ["" ("format string") w795 w853 w870 w878 w884] -> w785
              tunnel: w790 -> [_ w794 w841 w862 w877 w886]
              frame Default {
              }
              frame "Solve" {
                n397 = Variant To Data(type=T25 {"format string"="", "Measurement Index"=[]} ("output cluster"), Variant=w800) -> (data=w798:T25)  [unwired: 1 in, 1 out]
                n398 = Unbundle(w798) -> ("format string"=w797:string, "Measurement Index"=w796:i32[])
                n399 = case shown="\"\"" w797 {
                  tunnel: w796 -> [_ w809 w822 w835]
                  tunnel: ["-" w803 w816 w829] -> w795
                  tunnel: w794 -> [_ w802 w815 w828]
                  frame Default {
                  }
                  frame "" {
                    n400 = Number To Decimal String(number=w809) -> (decimal integer string=w808:string[])  [unwired: 1 in]
                    n401 = for {
                      tunnel: w808 -> [w813] mode=indexing
                      shift-right: [w814] -> w806
                      shift-left: "[ " ("String") -> [w810]
                      n402 = Concatenate Strings(w810, "M" ("string"), w813, " " ("String")) -> (w814:string)
                    }
                    n403 = Concatenate Strings(w802, "Resolver Mediciones -> " ("format string"), w806, "]" ("String")) -> (w803:string)
                  }
                  frame "Relev" {
                    n404 = Number To Decimal String(number=w822) -> (decimal integer string=w821:string[])  [unwired: 1 in]
                    n405 = for {
                      tunnel: w821 -> [w826] mode=indexing
                      shift-right: [w827] -> w819
                      shift-left: "[ " ("String") -> [w823]
                      n406 = Concatenate Strings(w823, "M" ("string"), w826, " " ("String")) -> (w827:string)
                    }
                    n407 = Concatenate Strings(w815, "Resolver Mediciones con relevamiento de Pieza Patron -> " ("format string"), w819, "]" ("String")) -> (w816:string)
                  }
                  frame "Mastering" {
                    n408 = Number To Decimal String(number=w835) -> (decimal integer string=w834:string[])  [unwired: 1 in]
                    n409 = for {
                      tunnel: w834 -> [w839] mode=indexing
                      shift-right: [w840] -> w832
                      shift-left: "[ " ("String") -> [w836]
                      n410 = Concatenate Strings(w836, "M" ("string"), w839, " " ("String")) -> (w840:string)
                    }
                    n411 = Concatenate Strings(w828, "Resolver Mediciones con Mastering -> " ("format string"), w832, "]" ("String")) -> (w829:string)
                  }
                }
              }
              frame "Mastering" {
                n412 = Variant To Data(type=T26 {"MAX(T) or MIN (F)?"=FALSE, "Mastering TDX Index"=[]} ("output cluster"), Variant=w856) -> (data=w855:T26)  [unwired: 1 in, 1 out]
                n413 = Unbundle(w855) -> ("MAX(T) or MIN (F)?"=w847:bool, "Mastering TDX Index"=w854:i32[])
                n414 = Number To Decimal String(number=w854) -> (decimal integer string=w852:string[])  [unwired: 1 in]
                n415 = for {
                  tunnel: w852 -> [w860] mode=indexing
                  shift-right: [w861] -> w850
                  shift-left: "[ " ("String") -> [w857]
                  n416 = Concatenate Strings(w857, "T" ("string"), w860, " " ("String")) -> (w861:string)
                }
                n417 = Select(t="MAXIMO" ("format string"), s=w847, f="MINIMO" ("format string")) -> (s? t:f=w843:string)
                n418 = Format Into String(format string="Tomar %s de los Transductores ->", w843) -> (resulting string=w842:string)  [unwired: 2 in, 1 out]
                n419 = Concatenate Strings(w841, w842, w850, "]" ("String")) -> (w853:string)
              }
              frame "Auto-Zero" {
                n420 = Variant To Data(type=i32[] [] ("Mastering TDX Index"), Variant=w871) -> (data=w863:i32[])  [unwired: 1 in, 1 out]
                n421 = Number To Decimal String(number=w863) -> (decimal integer string=w869:string[])  [unwired: 1 in]
                n422 = for {
                  tunnel: w869 -> [w875] mode=indexing
                  shift-right: [w876] -> w867
                  shift-left: "[ " ("String") -> [w872]
                  n423 = Concatenate Strings(w872, "T" ("string"), w875, " " ("String")) -> (w876:string)
                }
                n424 = Concatenate Strings(w862, "Calcular Zero de los Transductores ->" ("format string"), w867, "]" ("String")) -> (w870:string)
              }
              frame "Relev" {
                n425 = Variant To Data(type=0, Variant=w883) -> (data=w880:i32)  [unwired: 1 in, 1 out]
                n426 = Format Into String(format string="Calcular Relevamiento de Pieza Patron en Transductor T%d", w880) -> (resulting string=w879:string)  [unwired: 2 in, 1 out]
                n427 = Concatenate Strings(w877, w879) -> (w878:string)
              }
              frame "Scale Calibrate" {
                n428 = Concatenate Strings(w886, "Calcular Constantes de calibracion de Balanzas" ("format string")) -> (w884:string)
              }
            }
            n429 = Unbundle By Name(w788) -> ("MATH"=w787:string)
            n430 = Concatenate Strings(w787, w785, "\r\n") -> (w784:string)
            "MATH" <- w784
            n431 = Bundle By Name(cluster=w788, "MATH"=w784) -> (w789:T10)
          }
        }
      }
      frame "EXIT" {
      }
      frame "Init" {
        n432 = invoke on="HWSync 1" class="Str" method="Reinit To Default"(error in=w891) -> (error out=w903:errorcluster)  [unwired: 2 in, 2 out]
        n433 = invoke on="HWSync 2" class="Str" method="Reinit To Default"(error in=w891) -> (error out=w902:errorcluster)  [unwired: 2 in, 2 out]
        n434 = invoke on="HWSync 3" class="Str" method="Reinit To Default"(error in=w891) -> (error out=w901:errorcluster)  [unwired: 2 in, 2 out]
        n435 = invoke on="HWSync 4" class="Str" method="Reinit To Default"(error in=w891) -> (error out=w900:errorcluster)  [unwired: 2 in, 2 out]
        n436 = invoke on="HWSync 5" class="Str" method="Reinit To Default"(error in=w891) -> (error out=w899:errorcluster)  [unwired: 2 in, 2 out]
        n437 = invoke on="DO 1" class="Arr (strict)" method="Reinit To Default"(error in=w891) -> (error out=w898:errorcluster)  [unwired: 2 in, 2 out]
        n438 = invoke on="DO 2" class="Arr (strict)" method="Reinit To Default"(error in=w891) -> (error out=w897:errorcluster)  [unwired: 2 in, 2 out]
        n439 = invoke on="DO 3" class="Arr (strict)" method="Reinit To Default"(error in=w891) -> (error out=w896:errorcluster)  [unwired: 2 in, 2 out]
        n440 = invoke on="DO 4" class="Arr (strict)" method="Reinit To Default"(error in=w891) -> (error out=w895:errorcluster)  [unwired: 2 in, 2 out]
        n441 = invoke on="DO 5" class="Arr (strict)" method="Reinit To Default"(error in=w891) -> (error out=w894:errorcluster)  [unwired: 2 in, 2 out]
        n442 = Merge Errors(w903, w902, w901, w900, w899, w898, w897, w896, w895, w894) -> (w892:errorcluster)
        n443 = invoke on="HWAsync 1" class="Str" method="Reinit To Default"(error in=w892) -> (error out=w913:errorcluster)  [unwired: 2 in, 2 out]
        n444 = invoke on="HWAsync 2" class="Str" method="Reinit To Default"(error in=w892) -> (error out=w912:errorcluster)  [unwired: 2 in, 2 out]
        n445 = invoke on="HWAsync 3" class="Str" method="Reinit To Default"(error in=w892) -> (error out=w911:errorcluster)  [unwired: 2 in, 2 out]
        n446 = invoke on="HWAsync 4" class="Str" method="Reinit To Default"(error in=w892) -> (error out=w910:errorcluster)  [unwired: 2 in, 2 out]
        n447 = invoke on="HWAsync 5" class="Str" method="Reinit To Default"(error in=w892) -> (error out=w909:errorcluster)  [unwired: 2 in, 2 out]
        n448 = invoke on="HWAsync 6" class="Str" method="Reinit To Default"(error in=w892) -> (error out=w908:errorcluster)  [unwired: 2 in, 2 out]
        n449 = invoke on="HWAsync 7" class="Str" method="Reinit To Default"(error in=w892) -> (error out=w907:errorcluster)  [unwired: 2 in, 2 out]
        n450 = invoke on="HWAsync 8" class="Str" method="Reinit To Default"(error in=w892) -> (error out=w906:errorcluster)  [unwired: 2 in, 2 out]
        n451 = invoke on="HWAsync 9" class="Str" method="Reinit To Default"(error in=w892) -> (error out=w905:errorcluster)  [unwired: 2 in, 2 out]
        n452 = invoke on="HWAsync 10" class="Str" method="Reinit To Default"(error in=w892) -> (error out=w904:errorcluster)  [unwired: 2 in, 2 out]
        n453 = invoke on="MATH" class="Str" method="Reinit To Default"(error in=w892) -> (error out=w893:errorcluster)  [unwired: 2 in, 2 out]
        n454 = Merge Errors(w913, w912, w911, w910, w909, w908, w907, w906, w905, w904, w893) -> (w890:errorcluster)
      }
      frame "CONFIG" {
        # "\"CONFIG:<Tipo>:<Indice>\" ; <Config Data>"
        n455 = Generate User Event(user event=w918, event data cluster=w919, error in=w917) -> (error out=w916:errorcluster)  [unwired: 1 in, 1 out]
      }
    }
  }
  n456 = call "SeqLoop.vi"("SEQ STEP Display"=w51, "error in (no error)"=w56, "SEQ"=w58, "CORE"=w59, "WINFAS 2 Data Queue"=w57) -> ("error out"=w55:errorcluster)  [unwired: 6 in]
  n457 = Set Occurrence(w82) -> ()
  n458 = Merge Errors(w101, w55) -> (w98:errorcluster)
  n459 = call "Destroy All Message Queues.vi"("error in (no error)"=w98, "Message Queues Out"=w61) -> ("error out"=w63:errorcluster)  [unwired: 9 in]
  n460 = call "Destroy All Data Queues.vi"("Error In"=w63, "WINFAS 2 Data Queue.lvlib:All Data Queues Cluster"=w57) -> ("Error Out"=w62:errorcluster)  [unwired: 9 in]
  n461 = Release Notifier(notifier=w51, error in (no error)=w62) -> (error out=w84:errorcluster)  [unwired: 1 in, 2 out]
  n462 = property class="App"(error in=w84) -> ("App.Kind"=w89:T27)  [unwired: 1 in, 2 out]
  n463 = case shown="\"Run Time System\"" w89 {
    tunnel: [TRUE FALSE TRUE] -> w88
    tunnel: [w920 w934 w940] -> _
    frame "invalid app kind", Default {
      n464 = property class="VI"() -> (error out=w921:errorcluster, "Panel"=w931:refnum<vi>)  [unwired: 2 in, 1 out]
      n465 = property class="Pnl"(reference=w931, error in=w921) -> (error out=w922:errorcluster, "AllObjs[]"=w930:refnum<vi>[])  [unwired: 1 out]
      n466 = control-ref of="This VI"() -> (w928:refnum<vi>)
      n467 = Close Reference(reference=w930, error in (no error)=w922) -> (error out=w927:errorcluster)
      n468 = invoke class="VI" method="FP.Close"(reference=w928, error in=w927) -> (reference out=w926:refnum<vi>, error out=w925:errorcluster)  [unwired: 1 in, 1 out]
      n469 = invoke class="VI" method="Abort VI"(reference=w926, error in=w925) -> (reference out=w923:refnum<vi>, error out=w924:errorcluster)  [unwired: 1 in, 1 out]
      n470 = Close Reference(reference=w923, error in (no error)=w924) -> (error out=w932:errorcluster)
      n471 = control-ref of="This Application"() -> (w933:refnum<vi>)
      n472 = Close Reference(reference=w933, error in (no error)=w932) -> (error out=w920:errorcluster)
    }
    frame "Development System" {
      n473 = property class="VI"() -> (error out=w935:errorcluster, "Panel"=w939:refnum<vi>)  [unwired: 2 in, 1 out]
      n474 = property class="Pnl"(reference=w939, error in=w935) -> (error out=w936:errorcluster, "AllObjs[]"=w938:refnum<vi>[])  [unwired: 1 out]
      n475 = Close Reference(reference=w938, error in (no error)=w936) -> (error out=w934:errorcluster)
    }
    frame "Run Time System" {
      n476 = property class="VI"() -> (error out=w941:errorcluster, "Panel"=w951:refnum<vi>)  [unwired: 2 in, 1 out]
      n477 = property class="Pnl"(reference=w951, error in=w941) -> (error out=w942:errorcluster, "AllObjs[]"=w950:refnum<vi>[])  [unwired: 1 out]
      n478 = control-ref of="This VI"() -> (w948:refnum<vi>)
      n479 = Close Reference(reference=w950, error in (no error)=w942) -> (error out=w947:errorcluster)
      n480 = invoke class="VI" method="FP.Close"(reference=w948, error in=w947) -> (reference out=w946:refnum<vi>, error out=w945:errorcluster)  [unwired: 1 in, 1 out]
      n481 = invoke class="VI" method="Abort VI"(reference=w946, error in=w945) -> (reference out=w943:refnum<vi>, error out=w944:errorcluster)  [unwired: 1 in, 1 out]
      n482 = Close Reference(reference=w943, error in (no error)=w944) -> (error out=w952:errorcluster)
      n483 = control-ref of="This Application"() -> (w953:refnum<vi>)
      n484 = Close Reference(reference=w953, error in (no error)=w952) -> (error out=w940:errorcluster)
    }
  }
  n485 = Quit LabVIEW(quit? (T)=w88) -> ()
